vi "Filter Wheel GUI.vi"(9 "Standalone":bool=TRUE, 10 "Init Data":variant, 11 "Filter Wheel name":string="Default") -> ()   [LabVIEW 2024]
uses:
  Filter Wheel Arduino Control/Filter Wheel Arduino Command cluster.ctl
  typedefs/CC enum Operation Mode.ctl
  Filter Wheel Arduino Control/Filter Wheel Arduino Homing cluster.ctl
  Filter Wheel Object/Filter Wheel.lvclass
  Filter Wheel configuration.ctl
  Filter Wheel Object/Filter Wheel Details.ctl
  Subsystems/SS typedef cluster Instrument Command Queue Data.ctl
  Subsystems/SS cluster Data Queue type.ctl
  FW cmd Q Move Parameters.ctl
  <vilib>/Utility/miscctls.llb/LVRowAndColumnTypeDef.ctl
  FW cluster Status.ctl
  FW enum status.ctl
  Filter Wheel Object/Filter Wheel.lvclass/Filter Wheel.ctl
  hk-channel-class/hk-channel-class/HK Item/HK Channel Units and Setup.ctl
  hk-channel-class/hk-channel-class/HK Item/HK Channel enum Data Type.ctl
  hk-channel-class/hk-channel-class/HK Item/HK Item.lvclass
  hk-channel-class/hk-channel-class/HK Item/HK Channel cluster Telemetry Data.ctl
  FW cmd Q Move Position Parameters.ctl
  typedefs/CC cluster Alarm Data.ctl
  Filter Wheel Simulator/Filter Wheel Simulator.lvclass
  C:/Development/Prime-RIMAS/Filter Wheel/Filter Wheel Object/Filter Wheel.lvclass
  Filter Wheel Simulator/Filter Wheel Simulator.lvclass/Filter Wheel Simulator.ctl
  Filter Wheel Arduino Control/FW Arduino Control.lvclass
panel:
  out "Messages":string
  in  "Mode":T1
  in  "Tab Control":T2(tab)
  out "Wheel Name":string
  out "Moving Message":string="Filter Wheel Moving...."
  in  "Error":bool
  out "Homed":bool[](array[boolean])
  in  "Wheel To Home":u16(ring)
  in  "STOP":bool
  out "Connected":bool
  in  "Filter Wheel Displays":T3 {"Gauge 0" scale=0.0..3.0; "Gauge 4" scale=0.0..7.0; "Gauge 3" scale=0.0..5.0; "Gauge 2" scale=0.0..3.0; "Gauge 5" scale=0.0..32768.0; "Gauge 8" scale=0.0..32768.0; "Gauge 6" scale=0.0..32768.0; "Gauge 7" scale=0.0..32768.0}
  in  "Home":bool
  in  "Alarms?":bool=TRUE
  in  "Default Speed":u16=200 min=20 max=4000 step=10
  in  "Movement Parameters":T4
  in  "Sim Velocity (steps/sec)":i32
  in  "Connect":bool
  in  "Serial Port":refnum<visa-resource-name>="COM11"
  in  "Simulate":bool
  in  "Close":bool
  in  "Filter Wheel Table":cluster{i32[], "Dir":bool}[][](array[cluster])=[[{[], "Dir"=TRUE}, {[2800], "Dir"=TRUE}, {[2800, 2800], "Dir"=TRUE}, {[950, 1850], "Dir"=FALSE}], [{[2800], "Dir"=FALSE}, {[], "Dir"=TRUE}, {[2800], "Dir"=TRUE}, {[2800, 2800], "Dir"=TRUE}], [{[2800, 2800], "Dir"=FALSE}, {[2800], "Dir"=FALSE}, {[], "Dir"=TRUE}, {[2800], "Dir"=TRUE}], [{[2800, 2800], "Dir"=TRUE}, {[2800, 2800], "Dir"=FALSE}, {[2800], "Dir"=FALSE}, {[], "Dir"=TRUE}]]
  in  "Open Arduino Log":bool
  out "Moving":bool[](array[boolean])
  out "Last Move Positions":u32[](array[numeric])
  out "On the notch":bool[](array[boolean])
  in  "Filter Wheel Settings":T5={"Direction"=TRUE, "NUMBER OF  STEPS"=2900, "SPEED STEPS/SEC"=200, "ACC/DECEL STEPS/SEC^2"=4000, "Move mode"=0, "EN/DIS?"=TRUE, "delay before \nread (ms)"=750, "Timeout before \nstop (ms)"=13000} {"Move mode" items=["Relative steps ##", "Search switch"]; "ACC/DECEL STEPS/SEC^2" max=4000; "SPEED STEPS/SEC" min=20 max=4000 step=10}
  in  "MOTOR NUMBER":u8 max=3 step=1
  in  "Command Preview":string
  out "Response":string
  in  "Send Command":bool
  in  "Read":bool
  in  "Focus Offsets":string[][](table)
  in  "Restore Defaults":bool
  in  "Remove Pos":bool
  in  "Add Pos":bool
  in  "Save Button":bool
  in  "Remove Fw":bool
  in  "Add Fw":bool
  in  "Wheels":i32(listbox)
  in  "Positions":i32(listbox)
  # "Click for info"
  # "Enter the combined offset of each combination of filters."
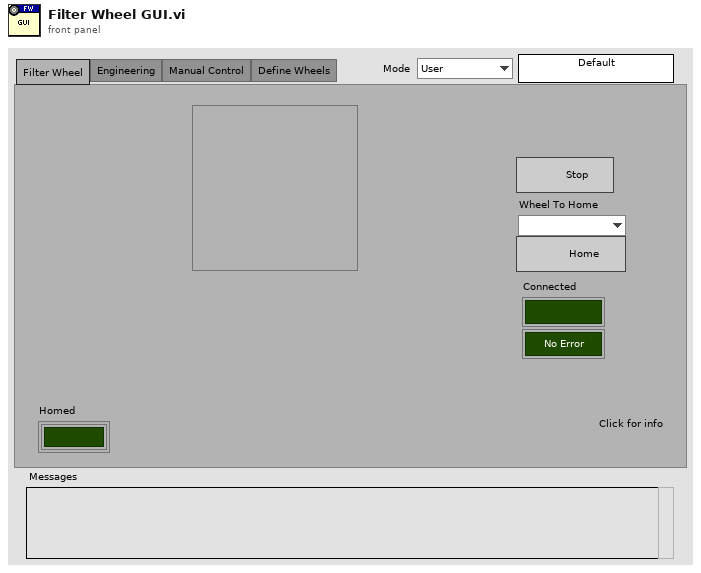
[diagram p1: front panel]
types:
  T1 = typedef "CC enum Operation Mode.ctl" = enum16{"User", "Engineering"}
  T2 = enum32{"Filter Wheel", "Engineering", "Manual Control", "Define Wheels"}
  T3 = cluster{"Gauge 0":i32, "Gauge 2":i32, "Gauge 3":i32, "Gauge 4":i32, "Gauge 5":i32, "Gauge 6":i32, "Gauge 7":i32, "Gauge 8":i32, "Position 0":i32, "Position 1":i32, "Position 2":i32, "Position 3":i32}
  T4 = typedef "Filter Wheel Arduino Homing cluster.ctl" = cluster{"Direction (F: CW)":bool, "Speed":i32, "Accel":i32, "Min Distance":i32, "Short Leg":i32, "Error Cnts":i32}
  T5 = typedef "Filter Wheel Arduino Command cluster.ctl" = cluster{"Direction":bool, "NUMBER OF  STEPS":u32, "SPEED STEPS/SEC":u16, "ACC/DECEL STEPS/SEC^2":u16, "Move mode":u16, "EN/DIS?":bool, "delay before \nread (ms)":u32, "Timeout before \nstop (ms)":u32}
  T6 = typedef "SS typedef cluster Instrument Command Queue Data.ctl" = cluster{"Cmd":string, "Parameters":variant}
  T7 = typedef "Filter Wheel.lvclass/Filter Wheel configuration.ctl" = cluster{"Num Wheels":i32, "Filters":T8[], "Invalid Combinations":i32[][], "Addr":refnum<visa-resource-name>, "Name":string, "Simulate":bool, "Homing Parameters":T4, "Default Speed":u16}
  T8 = typedef "Filter Wheel.lvclass/Filter Wheel Details.ctl" = cluster{"Names":string[], "Relative Position":i32[], "Wheel Name":string}
  T9 = typedef "FW cmd Q Move Parameters.ctl" = cluster{"Wheel ID":i32, "Position":i32}
  T10 = typedef "LVRowAndColumnTypeDef.ctl" = cluster{"Row":i32, "Column":i32}
  T11 = typedef "FW cluster Status.ctl" = cluster{"State":T12, "Positions":i32[], "Names":string[], "Notch":bool[], "Moving":bool[]}
  T12 = typedef "FW enum status.ctl" = enum16{"Initializing", "Moving", "Move Complete", "Error"}
  T13 = cluster{"state":refnum<user-event>, "Filter Wheel ref":refnum<class "Filter Wheel.lvclass">, "Filter Wheel Info":T7, "FW names":string[], "Pos Names":cluster{"Table":string[][]}[], "cmd q":refnum<queue>, "Cmd":T6, "Data Q":refnum<queue>, "Move":T9, "error":errorcluster, "next poll":timestamp, "FW refs":refnum<vi>[], "Wheel":i32, "Coords":T10, "Motor #":u8, "fw name":string, "Simulate":bool, "ch names":string[][], "FW Status":T11, "Error State":string, "Name":string, "Period":dbl}
  T14 = typedef "HK Item.lvclass/HK Channel Units and Setup.ctl" = cluster{"Unit Type":string, "Units":string, "Configuration":string, "Digits":i32, "Data Type":T15, "Exponential?":bool, "Source":string}
  T15 = typedef "HK Item.lvclass/HK Channel enum Data Type.ctl" = enum16{"Floating Point", "Integer", "Enum", "String", "Waveform", "File"}
  T16 = typedef "SS cluster Data Queue type.ctl" = cluster{"Source":string, "Type":string, "Data":variant}
  T17 = typedef "FW cmd Q Move Position Parameters.ctl" = cluster{"Position Names":string[]}
  T18 = enum32{"Page Enabled", "Page Disabled", "Page Disabled & Grayed"}
  T19 = typedef "CC cluster Alarm Data.ctl" = cluster{"Measured Value":dbl, "Alarm Low":dbl, "Alarm High":dbl, "Message":string, "Source":string}
  T20 = typedef "HK Item.lvclass/HK Channel cluster Telemetry Data.ctl" = cluster{"Ch Names":string[], "Ch Values":dbl[], "Timestamp":timestamp, "Data Type":T15}
  T21 = cluster{"Gauge 0":bool, "Gauge 2":bool, "Gauge 3":bool, "Gauge 4":bool, "Gauge 5":bool, "Gauge 6":bool, "Gauge 7":bool, "Gauge 8":bool, "Position 0":bool, "Position 1":bool, "Position 2":bool, "Position 3":bool}
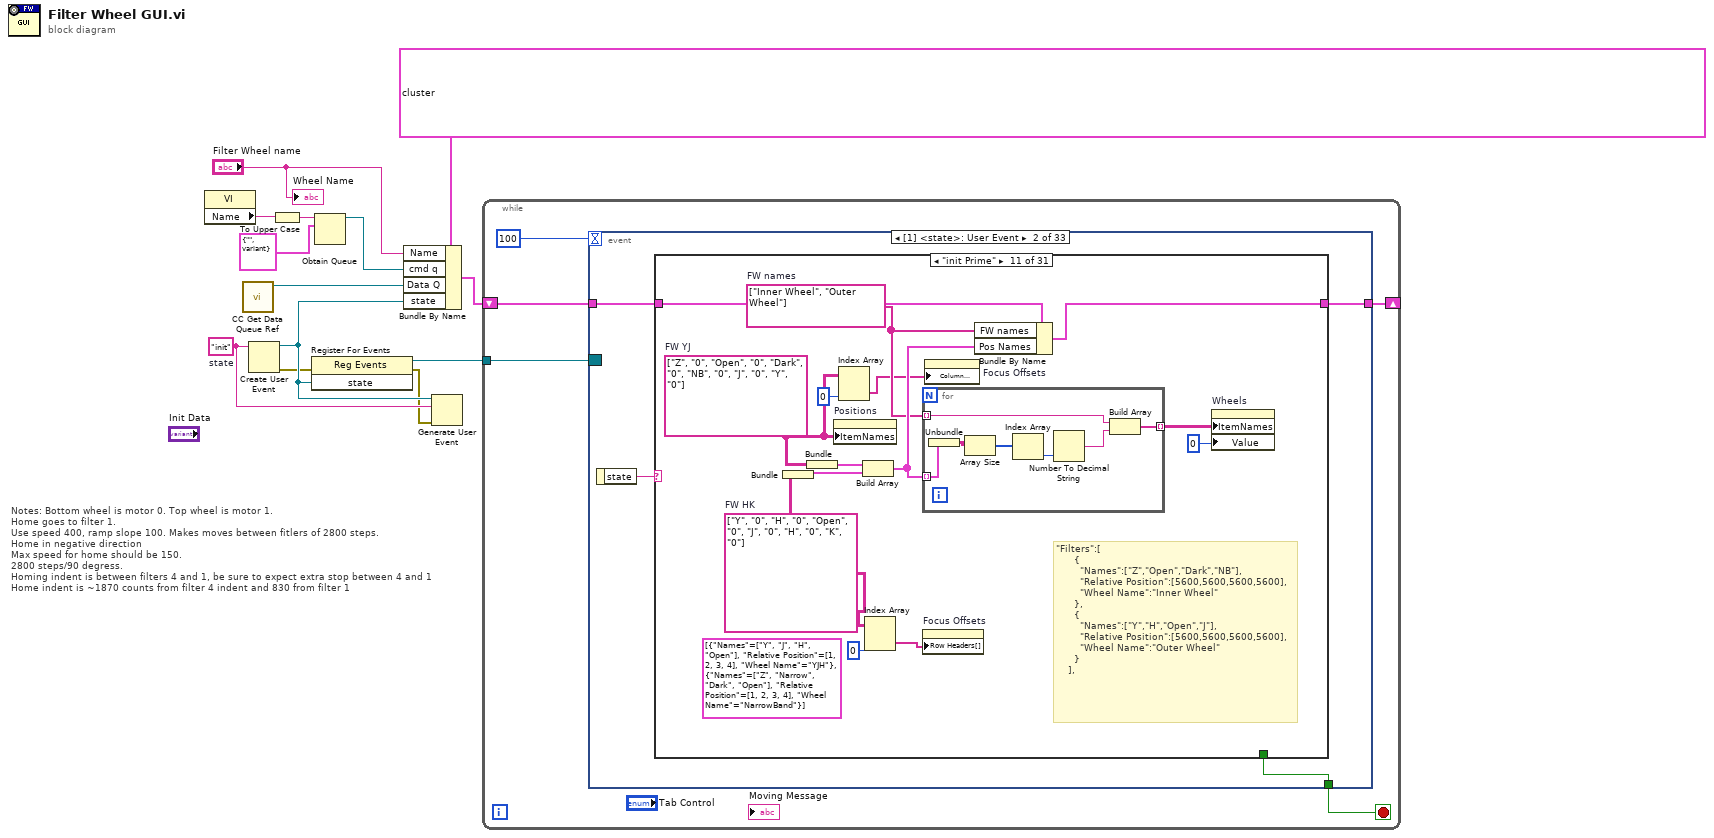
[diagram p0: block diagram]
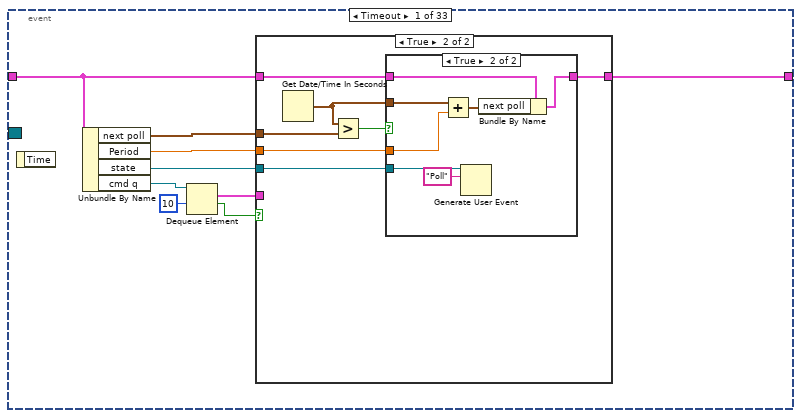
[diagram p2: hidden frame]
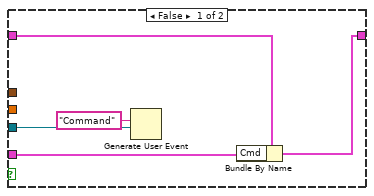
[diagram p3: hidden frame]
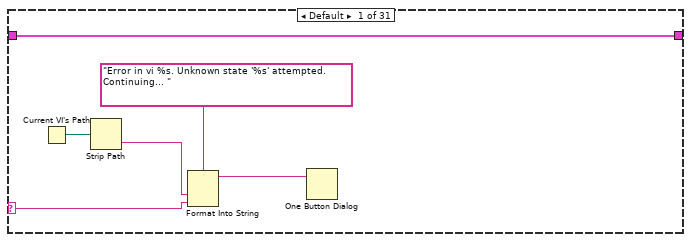
[diagram p5: hidden frame]
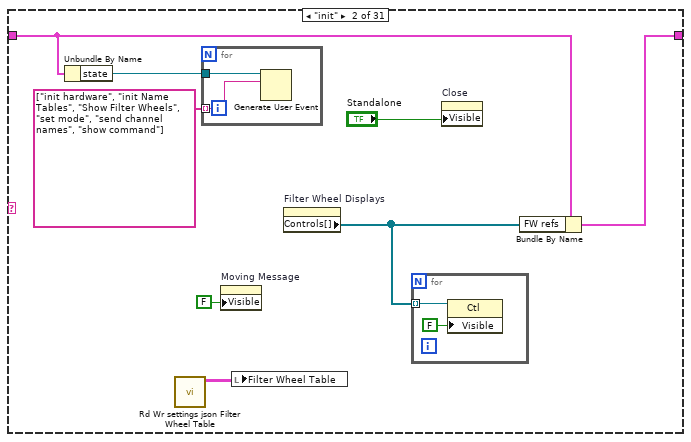
[diagram p6: hidden frame]
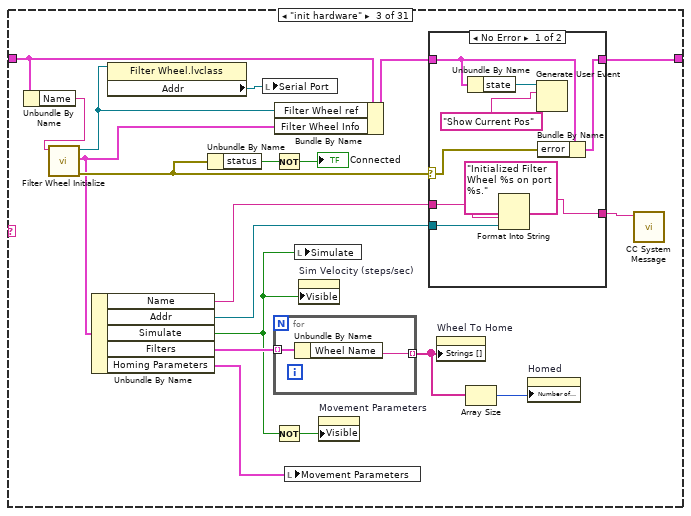
[diagram p7: hidden frame]
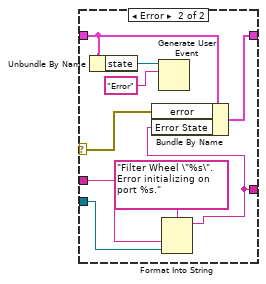
[diagram p8: hidden frame]
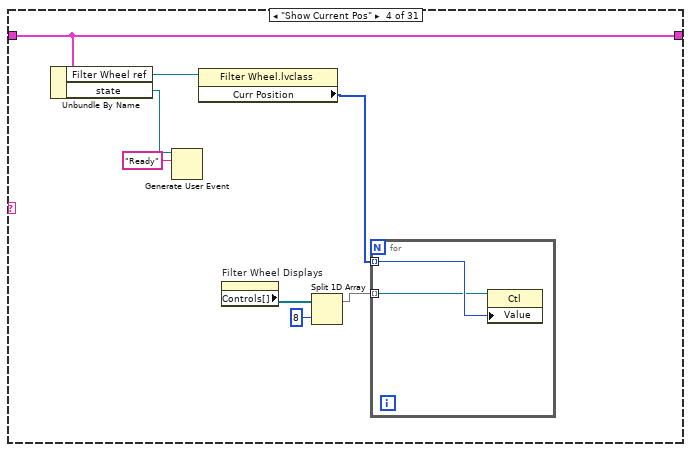
[diagram p9: hidden frame]
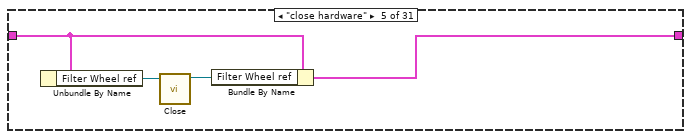
[diagram p10: hidden frame]
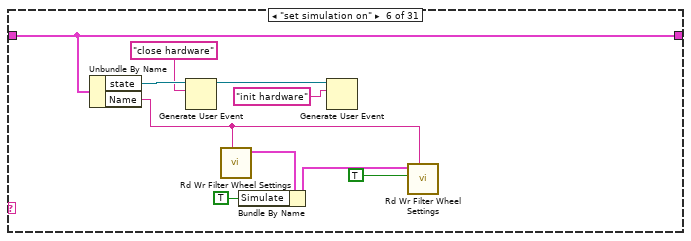
[diagram p11: hidden frame]
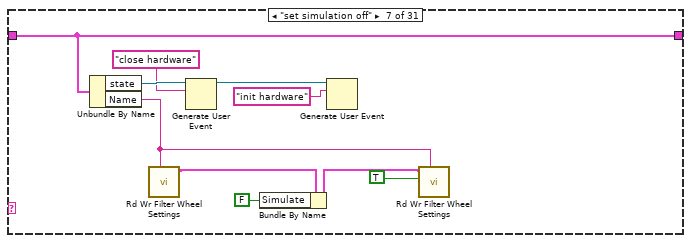
[diagram p12: hidden frame]
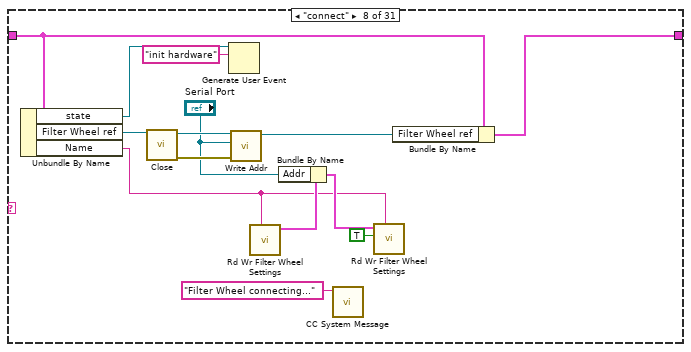
[diagram p13: hidden frame]
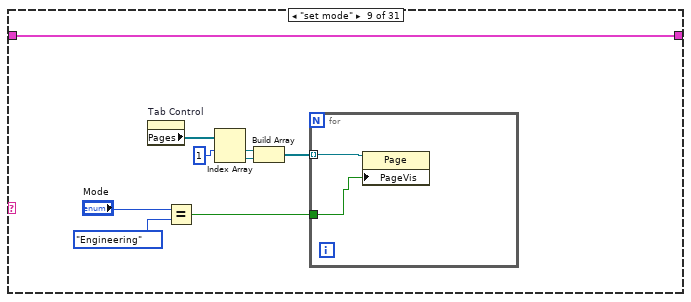
[diagram p14: hidden frame]
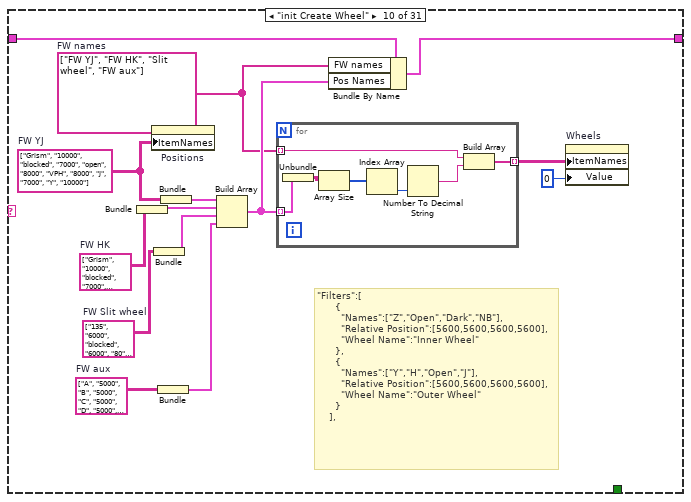
[diagram p15: hidden frame]
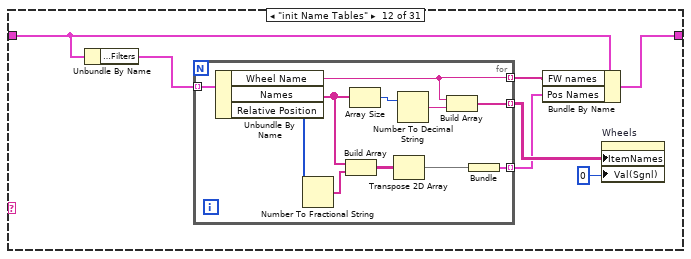
[diagram p16: hidden frame]
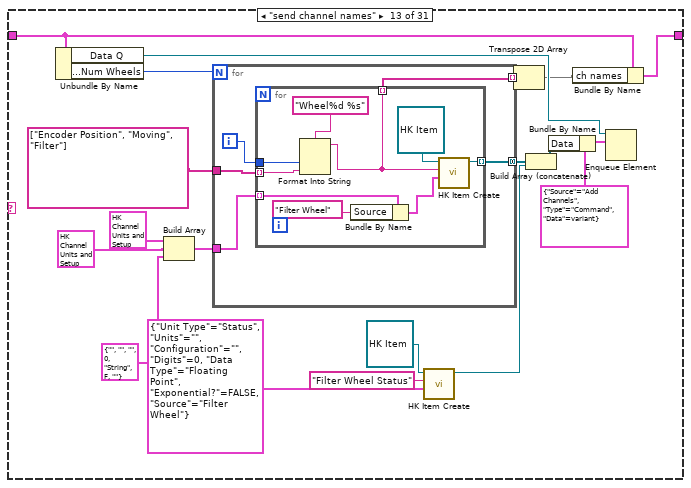
[diagram p17: hidden frame]
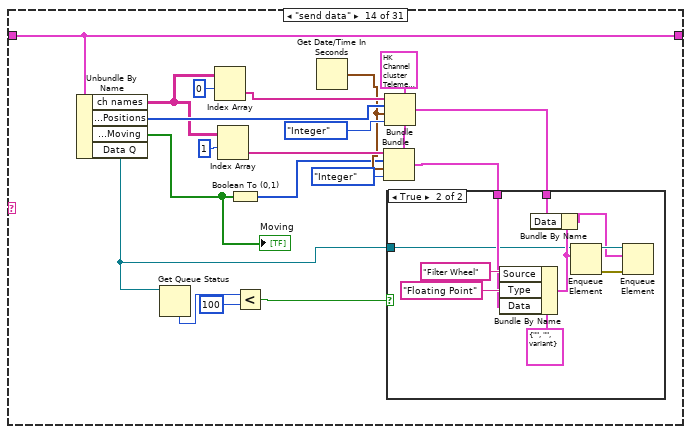
[diagram p18: hidden frame]
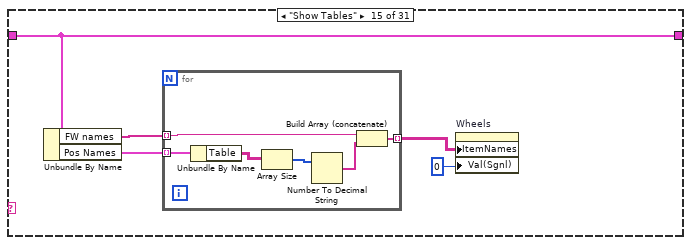
[diagram p20: hidden frame]
diagram:
  w9 = "init"  # state
  # "Notes: Bottom wheel is motor 0. Top wheel is motor 1.\nHome goes to filter 1. \nUse speed 400, ramp slope 100. Makes moves between fitlers of 2800 steps.\nHome in negative direction\nMax speed for home should be 150.\n2800 steps/90 degress.\nHoming indent is between filters 4 and 1, be sure to expect extra stop between 4 and 1\nHome indent is ~1870 counts from filter 4 indent and 830 from filter 1"
  n1 = property class="VI"() -> ("Name"=w5:string)  [unwired: 2 in, 2 out]
  n2 = call "CC Get Data Queue Ref.vi"() -> ("Data Q"=w6:refnum<queue>)  [unwired: 10 in, 1 out]
  n3 = Create User Event(user event datatype=w9) -> (user event=w11:refnum<user-event>, error out=w7:errorcluster)  [unwired: 1 in]
  n4 = To Upper Case(1:w5) -> (0:w4:string)
  n5 = register-events(error in=w7, w11) -> (reference out=w10:refnum<event-registration>, error out=w8:errorcluster)  [unwired: 1 in]
  n6 = Obtain Queue(name (unnamed)=w4, element data type=T6 {"Cmd"="", "Parameters"=variant}) -> (queue out=w2:refnum<queue>)  [unwired: 3 in, 2 out]
  n7 = Bundle By Name(cluster=T13 {"state"=refnum, "Filter Wheel ref"=refnum, "Filter Wheel Info"={"Num Wheels"=0, "Filters"=[], "Invalid Combinations"=[], "Addr"="", "Name"="", "Simulate"=FALSE, "Homing Parameters"={"Direction (F: CW)"=TRUE, "Speed"=150, "Accel"=400, "Min Distance"=2700, "Short Leg"=0, "Error Cnts"=0}, "Default Speed"=1000}, "FW names"=["FW YJ", "FW HK", "Slit wheel", "FW aux"], "Pos Names"=[], "cmd q"=refnum, "Cmd"={"Cmd"="", "Parameters"=variant}, "Data Q"=refnum, "Move"={"Wheel ID"=0, "Position"=0}, "error"={"status"=FALSE, "code"=0, "source"=""}, "next poll"=timestamp(0 s since 1904-01-01), "FW refs"=[], "Wheel"=0, "Coords"={"Row"=0, "Column"=0}, "Motor #"=0, "fw name"="", "Simulate"=TRUE, "ch names"=[], "FW Status"={"State"=enum."Move Complete", "Positions"=[], "Names"=[], "Notch"=[], "Moving"=[FALSE, FALSE]}, "Error State"="", "Name"="PRIME", "Period"=1.0}, "Name"="Filter Wheel name", "cmd q"=w2, "Data Q"=w6, "state"=w11) -> (w12:T13)
  n8 = Generate User Event(user event=w11, event data cluster=w9, error in=w8) -> ()  [unwired: 1 in, 2 out]
  n9 = while {
    tunnel: w10 -> [w18]
    shift-right: [w17] -> _
    shift-left: w12 -> [w14]
    stop <- w16 stop-if-true
    n10 = event shown="[1] <state>: User Event" {
      selector: w18 -> [_ _ _ _ _ _ _ _ _ _ _ _ _ _ _ _ _ _ _ _ _ _ _ _ _ _ _ _ _ _ _ _ _]
      dyn-events: _ -> [_ _ _ _ _ _ _ _ _ _ _ _ _ _ _ _ _ _ _ _ _ _ _ _ _ _ _ _ _ _ _ _ _]
      timeout: 100 -> [_ _ _ _ _ _ _ _ _ _ _ _ _ _ _ _ _ _ _ _ _ _ _ _ _ _ _ _ _ _ _ _ _]
      tunnel: w14 -> [w22 w50 w587 w589 w598 w604 w607 w610 w612 w634 w641 w650 w656 w657 w672 w675 w678 w679 w684 w687 w696 w700 w706 w713 w718 w734 w756 w765 w771 w794 w805 w825 w829]
      tunnel: [w21 w49 w587 w588 w598 w604 w607 w610 w615 w635 w642 w650 w656 w658 w672 w675 w678 w680 w684 w687 w697 w701 w707 w714 w719 w735 w757 w766 w772 w795 w806 w825 w829] -> w17
      tunnel: [_ w48 _ _ _ _ _ _ _ _ _ _ _ _ _ _ _ _ _ _ _ _ _ _ _ _ _ _ _ _ _ _ _] -> w16
      event Timeout {
        n11 = event-data() -> ()  [unwired: 1 in, 1 out]
        n12 = Unbundle By Name(w22) -> ("next poll"=w20:timestamp, "Period"=w19:dbl, "state"=w23:refnum<user-event>, "cmd q"=w27:refnum<queue>)
        n13 = Dequeue Element(queue=w27, timeout in ms (-1)=10) -> (element=w24:T6, timed out?=w25:bool)  [unwired: 1 in, 2 out]
        n14 = case shown="True" w25 {
          tunnel: w24 -> [w29 _]
          tunnel: w23 -> [w32 w36]
          tunnel: w22 -> [w30 w37]
          tunnel: [w28 w34] -> w21
          tunnel: w20 -> [_ w39]
          tunnel: w19 -> [_ w33]
          frame False {
            n15 = Generate User Event(user event=w32, event data cluster="Command" ("event data")) -> ()  [unwired: 2 in, 2 out]
            n16 = Bundle By Name(cluster=w30, "Cmd"=w29) -> (w28:T13)
          }
          frame True {
            n17 = Get Date/Time In Seconds() -> (seconds since 1Jan1904=w35:timestamp)
            n18 = Greater?(x=w35, y=w39) -> (0:w38:bool)
            n19 = case shown="True" w38 {
              tunnel: w37 -> [w40 w47]
              tunnel: w36 -> [_ w46]
              tunnel: w35 -> [_ w45]
              tunnel: [w40 w43] -> w34
              tunnel: w33 -> [_ w41]
              frame False {
              }
              frame True {
                n20 = Add(x=w45, y=w41) -> (x+y=w44:timestamp)
                n21 = Generate User Event(user event=w46, event data cluster="Poll" ("event data")) -> ()  [unwired: 2 in, 2 out]
                n22 = Bundle By Name(cluster=w47, "next poll"=w44) -> (w43:T13)
              }
            }
          }
        }
      }
      event User Event {
        n23 = event-data() -> ("state"=w51:string)  [unwired: 1 in]
        n24 = case shown="\"init Prime\"" w51 {
          selector: w51 -> [w56 _ _ _ _ _ _ _ _ _ _ _ _ _ _ _ _ _ _ _ _ _ _ _ _ _ _ _ _ _ _]
          tunnel: w50 -> [w52 w64 w75 w116 w119 w131 w141 w152 w165 w168 w195 w214 w235 w279 w294 w312 w328 w337 w379 w437 w460 w488 w504 w517 w533 w541 w548 w555 w560 w581 w584]
          tunnel: [w52 w65 w87 w116 w120 w131 w141 w153 w165 w169 w196 w215 w236 w279 w294 w312 w328 w338 w388 w438 w478 w487 w505 w518 w534 w542 w548 w555 w561 w581 w584] -> w49
          tunnel: [_ _ _ _ _ _ _ _ _ _ _ _ _ _ _ _ _ _ _ _ _ _ _ _ _ _ _ _ _ _ TRUE] -> w48
          frame Default {
            n25 = Current VI's Path() -> (path=w55:path)
            n26 = Strip Path(path=w55) -> (name=w54:string)  [unwired: 1 out]
            n27 = Format Into String(format string="Error in vi %s. Unknown state '%s' attempted. Continuing... ", w54, w56) -> (resulting string=w53:string)  [unwired: 2 in, 1 out]
            n28 = One Button Dialog(message=w53) -> ()  [unwired: 1 in, 1 out]
          }
          frame "init" {
            n29 = Unbundle By Name(w64) -> ("state"=w63:refnum<user-event>)
            n30 = call "Rd Wr settings json Filter Wheel Table.vi"() -> ("Filter Wheel Table"=w58:cluster{i32[], bool}[][])  [unwired: 10 in, 1 out]
            n31 = for {
              tunnel: w63 -> [w69]
              tunnel: string[] ["init hardware", "init Name Tables", "Show Filter Wheels", "set mode", "send channel names", "show command"] -> [w68] mode=indexing
              n32 = Generate User Event(user event=w69, event data cluster=w68) -> ()  [unwired: 2 in, 2 out]
            }
            n33 = property on="Moving Message" class="Str"("Visible"=FALSE) -> ()  [unwired: 2 in, 2 out]
            n34 = local write "Filter Wheel Table"(w58) -> ()
            n35 = property on="Filter Wheel Displays" class="Clust (strict)"() -> ("Controls[]"=w60:refnum<vi>[])  [unwired: 2 in, 2 out]
            n36 = for {
              tunnel: w60 -> [w67] mode=indexing
              n37 = property class="Ctl"(reference=w67, "Visible"=FALSE) -> ()  [unwired: 1 in, 2 out]
            }
            n38 = property on="Close" class="Bool"("Visible"="Standalone") -> ()  [unwired: 2 in, 2 out]
            n39 = Bundle By Name(cluster=w64, "FW refs"=w60) -> (w65:T13)
          }
          frame "init hardware" {
            n40 = Unbundle By Name(w75) -> ("Name"=w74:string)
            n41 = call "Filter Wheel Initialize.vi"("Wheel Name"=w74) -> ("error out"=w86:errorcluster, "Filter Wheel Info"=w83:T7, "Filter Wheel.lvclass"=w71:refnum<class "Filter Wheel.lvclass">)  [unwired: 8 in]
            n42 = Unbundle By Name(w83) -> ("Name"=w82:string, "Addr"=w81:refnum<visa-resource-name>, "Simulate"=w72:bool, "Filters"=w79:T8[], "Homing Parameters"=w78:T4)
            n43 = property class="Filter Wheel.lvclass"(reference=w71) -> ("Addr"=w70:refnum<visa-resource-name>)  [unwired: 1 in, 2 out]
            n44 = Unbundle By Name(w86) -> ("status"=w85:bool)
            n45 = local write "Serial Port"(w70) -> ()
            n46 = Not(x=w85) -> (.not. x?=→"Connected":bool)
            n47 = for {
              tunnel: [w89] -> w77 mode=indexing
              tunnel: w79 -> [w90] mode=indexing
              n48 = Unbundle By Name(w90) -> ("Wheel Name"=w89:string)
            }
            n49 = Not(x=w72) -> (.not. x?=w73:bool)
            n50 = Bundle By Name(cluster=w75, "Filter Wheel ref"=w71, "Filter Wheel Info"=w83) -> (w88:T13)
            n51 = local write "Movement Parameters"(w78) -> ()
            n52 = local write "Simulate"(w72) -> ()
            n53 = property on="Sim Velocity (steps/sec)" class="DigNum (strict)"("Visible"=w72) -> ()  [unwired: 2 in, 2 out]
            n54 = property on="Movement Parameters" class="Clust (strict)"("Visible"=w73) -> ()  [unwired: 2 in, 2 out]
            n55 = case shown="No Error" w86 {
              selector: w86 -> [w93 w107]
              tunnel: [w92 w106] -> w87
              tunnel: w88 -> [w91 w105]
              tunnel: w82 -> [w98 w102]
              tunnel: w81 -> [w97 w101]
              tunnel: [w96 w100] -> w80
              frame No Error {
                n56 = Unbundle By Name(w91) -> ("state"=w94:refnum<user-event>)
                n57 = Format Into String(format string="Initialized Filter Wheel %s on port %s.", w98, w97) -> (resulting string=w96:string)  [unwired: 2 in, 1 out]
                n58 = Generate User Event(user event=w94, event data cluster="Show Current Pos" ("event data")) -> ()  [unwired: 2 in, 2 out]
                n59 = Bundle By Name(cluster=w91, "error"=w93) -> (w92:T13)
              }
              frame Error {
                n60 = Unbundle By Name(w105) -> ("state"=w104:refnum<user-event>)
                n61 = Generate User Event(user event=w104, event data cluster="Error" ("event data")) -> ()  [unwired: 2 in, 2 out]
                n62 = Format Into String(format string="Filter Wheel \"%s\". Error initializing on port %s.", w102, w101) -> (resulting string=w100:string)  [unwired: 2 in, 1 out]
                n63 = Bundle By Name(cluster=w105, "error"=w107, "Error State"=w100) -> (w106:T13)
              }
            }
            n64 = property on="Wheel To Home" class="Ring (strict)"("Strings []"=w77) -> ()  [unwired: 2 in, 2 out]
            n65 = Array Size(array=w77) -> (size(s)=w76:i32)
            n66 = property on="Homed" class="Arr (strict)"("Number of Columns"=w76) -> ()  [unwired: 2 in, 2 out]
            n67 = call "CC System Message.vi"("Message"=w80) -> ()  [unwired: 10 in, 1 out]
          }
          frame "Show Current Pos" {
            n68 = Unbundle By Name(w116) -> ("Filter Wheel ref"=w115:refnum<class "Filter Wheel.lvclass">, "state"=w114:refnum<user-event>)
            n69 = Generate User Event(user event=w114, event data cluster="Ready" ("event data")) -> ()  [unwired: 2 in, 2 out]
            n70 = property class="Filter Wheel.lvclass"(reference=w115) -> ("Curr Position"=w110:i32[])  [unwired: 1 in, 2 out]
            n71 = property on="Filter Wheel Displays" class="Clust (strict)"() -> ("Controls[]"=w112:refnum<vi>[])  [unwired: 2 in, 2 out]
            n72 = Split 1D Array(array=w112, index=8) -> (first subarray=w109:refnum<vi>[])  [unwired: 1 out]
            n73 = for {
              tunnel: w110 -> [w118] mode=indexing
              tunnel: w109 -> [w117] mode=indexing
              n74 = property class="Ctl"(reference=w117, "Value"=w118) -> ()  [unwired: 1 in, 2 out]
            }
          }
          frame "close hardware" {
            n75 = Unbundle By Name(w119) -> ("Filter Wheel ref"=w122:refnum<class "Filter Wheel.lvclass">)
            n76 = call-dynamic "Close.vi"("Filter Wheel in"=w122) -> ("Filter Wheel out"=w121:refnum<class "Filter Wheel.lvclass">)  [unwired: 9 in, 1 out]
            n77 = Bundle By Name(cluster=w119, "Filter Wheel ref"=w121) -> (w120:T13)
          }
          frame "set simulation on" {
            n78 = Unbundle By Name(w131) -> ("state"=w130:refnum<user-event>, "Name"=w123:string)
            n79 = Generate User Event(user event=w130, event data cluster="close hardware" ("event data")) -> (user event out=w129:refnum<user-event>)  [unwired: 2 in, 1 out]
            n80 = call "Rd Wr Filter Wheel Settings.vi"("Wheel Name"=w123) -> ("Filter Wheel Settings"=w126:T7)  [unwired: 9 in, 1 out]
            n81 = Bundle By Name(cluster=w126, "Simulate"=TRUE) -> (w125:T7)
            n82 = Generate User Event(user event=w129, event data cluster="init hardware" ("event data")) -> ()  [unwired: 2 in, 2 out]
            n83 = call "Rd Wr Filter Wheel Settings.vi"("Wheel Name"=w123, "Write? (F:Read)"=TRUE, "Filter Wheel Settings"=w125) -> ()  [unwired: 7 in, 2 out]
          }
          frame "set simulation off" {
            n84 = Unbundle By Name(w141) -> ("state"=w140:refnum<user-event>, "Name"=w133:string)
            n85 = call "Rd Wr Filter Wheel Settings.vi"("Wheel Name"=w133) -> ("Filter Wheel Settings"=w136:T7)  [unwired: 9 in, 1 out]
            n86 = Generate User Event(user event=w140, event data cluster="close hardware" ("event data")) -> (user event out=w139:refnum<user-event>)  [unwired: 2 in, 1 out]
            n87 = Bundle By Name(cluster=w136, "Simulate"=FALSE) -> (w135:T7)
            n88 = Generate User Event(user event=w139, event data cluster="init hardware" ("event data")) -> ()  [unwired: 2 in, 2 out]
            n89 = call "Rd Wr Filter Wheel Settings.vi"("Wheel Name"=w133, "Write? (F:Read)"=TRUE, "Filter Wheel Settings"=w135) -> ()  [unwired: 7 in, 2 out]
          }
          frame "connect" {
            n90 = Unbundle By Name(w152) -> ("state"=w150:refnum<user-event>, "Filter Wheel ref"=w156:refnum<class "Filter Wheel.lvclass">, "Name"=w143:string)
            n91 = call-dynamic "Close.vi"("Filter Wheel in"=w156) -> ("error out"=w154:errorcluster, "Filter Wheel out"=w155:refnum<class "Filter Wheel.lvclass">)  [unwired: 9 in]
            n92 = Generate User Event(user event=w150, event data cluster="init hardware" ("event data")) -> ()  [unwired: 2 in, 2 out]
            n93 = call "Write Addr.vi"("error in (no error)"=w154, "Addr"="Serial Port", "Filter Wheel in"=w155) -> ("Filter Wheel out"=w151:refnum<class "Filter Wheel.lvclass">)  [unwired: 7 in, 1 out]
            n94 = call "Rd Wr Filter Wheel Settings.vi"("Wheel Name"=w143) -> ("Filter Wheel Settings"=w148:T7)  [unwired: 9 in, 1 out]
            n95 = Bundle By Name(cluster=w148, "Addr"="Serial Port") -> (w146:T7)
            n96 = call "CC System Message.vi"("Message"="Filter Wheel connecting...") -> ()  [unwired: 10 in, 1 out]
            n97 = call "Rd Wr Filter Wheel Settings.vi"("Wheel Name"=w143, "Write? (F:Read)"=TRUE, "Filter Wheel Settings"=w146) -> ()  [unwired: 7 in, 2 out]
            n98 = Bundle By Name(cluster=w152, "Filter Wheel ref"=w151) -> (w153:T13)
          }
          frame "set mode" {
            n99 = property on="Tab Control" class="TabCtl (strict)"() -> ("Pages"=w164:refnum<vi>[])  [unwired: 2 in, 2 out]
            n100 = Equal?(x="Mode", y=CC_enum_Operation_Mode."Engineering") -> (x = y?=w157:bool)
            n101 = Index Array(array=w164, index #1=1 ("index")) -> (element #1=w162:refnum<vi>, element #2=w161:refnum<vi>)  [unwired: 1 in]
            n102 = Build Array(w162, w161) -> (w160:refnum<vi>[])
            n103 = for {
              tunnel: w160 -> [w167] mode=indexing
              tunnel: w157 -> [w166]
              n104 = property class="Page"(reference=w167, "PageVis"=w166) -> ()  [unwired: 1 in, 2 out]
            }
          }
          frame "init Create Wheel" {
            w170 = string[] ["FW YJ", "FW HK", "Slit wheel", "FW aux"]  # FW names
            w178 = string[][] [["Grism", "10000"], ["blocked", "7000"], ["open", "8000"], ["VPH", "8000"], ["J", "7000"], ["Y", "10000"]]  # FW YJ
            w181 = string[][] [["Grism", "10000"], ["blocked", "7000"], ["open", "8000"], ["VPH", "8000"], ["H", "7000"], ["K", "10000"]]  # FW HK
            w173 = string[][] [["135", "6000"], ["blocked", "6000"], ["80", "7000"], ["open 1", "7000"], ["250", "7000"], ["open", "7000"]]  # FW Slit wheel
            w180 = string[][] [["A", "5000"], ["B", "5000"], ["C", "5000"], ["D", "5000"], ["E", "5000"], ["F", "5000"], ["G", "5000"], ["H", "5000"]]  # FW aux
            # "\"Filters\":[\n      {\n        \"Names\":[\"Z\",\"Open\",\"Dark\",\"NB\"],\n        \"Relative Position\":[5600,5600,5600,5600],\n        \"Wheel Name\":\"Inner Wheel\"\n      },\n      {\n        \"Names\":[\"Y\",\"H\",\"Open\",\"J\"],\n        \"Relative Position\":[5600,5600,5600,5600],\n        \"Wheel Name\":\"Outer Wheel\"\n      }\n    ],"
            n105 = Bundle("FW HK"=w181) -> (w175:cluster{"FW HK":string[][]})  [unwired: 1 in]
            n106 = property on="Positions" class="MCListbox (strict)"("ItemNames"=w178) -> ()  [unwired: 2 in, 2 out]
            n107 = Bundle("FW Slit wheel"=w173) -> (w174:cluster{"FW Slit wheel":string[][]})  [unwired: 1 in]
            n108 = Bundle("FW aux"=w180) -> (w172:cluster{"FW aux":string[][]})  [unwired: 1 in]
            n109 = Bundle("FW YJ"=w178) -> (w176:cluster{"FW YJ":string[][]})  [unwired: 1 in]
            n110 = Build Array(w176, w175, w174, w172) -> (w171:cluster{"FW aux":string[][]}[])
            n111 = for {
              tunnel: w171 -> [w188] mode=indexing
              tunnel: w170 -> [w184] mode=indexing
              tunnel: [w183] -> w179 mode=indexing
              n112 = Unbundle(w188) -> ("FW aux"=w182:string[][])
              n113 = Array Size(array=w182) -> (size(s)=w187:i32[])
              n114 = Index Array(array=w187) -> (element=w186:i32)  [unwired: 1 in]
              n115 = Number To Decimal String(number=w186) -> (decimal integer string=w185:string)  [unwired: 1 in]
              n116 = Build Array(w184, w185) -> (w183:string[])
            }
            n117 = Bundle By Name(cluster=w168, "FW names"=w170, "Pos Names"=w171) -> (w169:T13)
            n118 = property on="Wheels" class="MCListbox (strict)"("ItemNames"=w179, "Value"=0 ("Wheels")) -> ()  [unwired: 2 in, 2 out]
          }
          frame "init Prime" {
            (unwired) T8[] [{"Names"=["Y", "J", "H", "Open"], "Relative Position"=[1, 2, 3, 4], "Wheel Name"="YJH"}, {"Names"=["Z", "Narrow", "Dark", "Open"], "Relative Position"=[1, 2, 3, 4], "Wheel Name"="NarrowBand"}] ("Filter Wheel Info.Filters")
            w197 = string[] ["Inner Wheel", "Outer Wheel"]  # FW names
            w194 = string[][] [["Z", "0"], ["Open", "0"], ["Dark", "0"], ["NB", "0"], ["J", "0"], ["Y", "0"]]  # FW YJ
            w191 = string[][] [["Y", "0"], ["H", "0"], ["Open", "0"], ["J", "0"], ["H", "0"], ["K", "0"]]  # FW HK
            # "\"Filters\":[\n      {\n        \"Names\":[\"Z\",\"Open\",\"Dark\",\"NB\"],\n        \"Relative Position\":[5600,5600,5600,5600],\n        \"Wheel Name\":\"Inner Wheel\"\n      },\n      {\n        \"Names\":[\"Y\",\"H\",\"Open\",\"J\"],\n        \"Relative Position\":[5600,5600,5600,5600],\n        \"Wheel Name\":\"Outer Wheel\"\n      }\n    ],"
            n119 = Bundle("FW HK"=w191) -> (w199:cluster{"FW HK":string[][]})  [unwired: 1 in]
            n120 = Bundle("FW YJ"=w194) -> (w200:cluster{"FW YJ":string[][]})  [unwired: 1 in]
            n121 = property on="Positions" class="MCListbox (strict)"("ItemNames"=w194) -> ()  [unwired: 2 in, 2 out]
            n122 = Index Array(array=w194, index (col)=0 ("disabled index (col)")) -> (element=w192:string[])  [unwired: 1 in]
            n123 = Build Array(w200, w199) -> (w198:cluster{"FW HK":string[][]}[])
            n124 = Index Array(array=w191, index (col)=0 ("disabled index (col)")) -> (element=w189:string[])  [unwired: 1 in]
            n125 = for {
              tunnel: w198 -> [w209] mode=indexing
              tunnel: w197 -> [w205] mode=indexing
              tunnel: [w204] -> w202 mode=indexing
              n126 = Unbundle(w209) -> ("FW HK"=w203:string[][])
              n127 = Array Size(array=w203) -> (size(s)=w208:i32[])
              n128 = Index Array(array=w208) -> (element=w207:i32)  [unwired: 1 in]
              n129 = Number To Decimal String(number=w207) -> (decimal integer string=w206:string)  [unwired: 1 in]
              n130 = Build Array(w205, w206) -> (w204:string[])
            }
            n131 = property on="Focus Offsets" class="Tbl (strict)"("Row Headers[]"=w189) -> ()  [unwired: 2 in, 2 out]
            n132 = property on="Focus Offsets" class="Tbl (strict)"("Column Headers[]"=w192) -> ()  [unwired: 2 in, 2 out]
            n133 = Bundle By Name(cluster=w195, "FW names"=w197, "Pos Names"=w198) -> (w196:T13)
            n134 = property on="Wheels" class="MCListbox (strict)"("ItemNames"=w202, "Value"=0 ("Wheels")) -> ()  [unwired: 2 in, 2 out]
          }
          frame "init Name Tables" {
            n135 = Unbundle By Name(w214) -> ("Filter Wheel Info.Filters"=w213:T8[])
            n136 = for {
              tunnel: w213 -> [w227] mode=indexing
              tunnel: [w224] -> w212 mode=indexing
              tunnel: [w223] -> w211 mode=indexing
              tunnel: [w218] -> w210 mode=indexing
              n137 = Unbundle By Name(w227) -> ("Wheel Name"=w224:string, "Names"=w220:string[], "Relative Position"=w222:i32[])
              n138 = Number To Fractional String(number=w222) -> (F-format string=w221:string[])  [unwired: 3 in]
              n139 = Build Array(w220, w221) -> (w219:string[][])
              n140 = Array Size(array=w220) -> (size(s)=w226:i32)
              n141 = Transpose 2D Array(2D array=w219) -> (transposed array=w217:string[][])
              n142 = Number To Decimal String(number=w226) -> (decimal integer string=w225:string)  [unwired: 1 in]
              n143 = Build Array(w224, w225) -> (w223:string[])
              n144 = Bundle(w217) -> (w218:cluster{string[][]})  [unwired: 1 in]
            }
            n145 = Bundle By Name(cluster=w214, "FW names"=w212, "Pos Names"=w210) -> (w215:T13)
            n146 = property on="Wheels" class="MCListbox (strict)"("ItemNames"=w211, "Val(Sgnl)"=0 ("Wheels")) -> ()  [unwired: 2 in, 2 out]
          }
          frame "send channel names" {
            n147 = Unbundle By Name(w235) -> ("Data Q"=w239:refnum<queue>, "Filter Wheel Info.Num Wheels"=w238:i32)
            n148 = Build Array(T14 {"Unit Type"="", "Units"="Counts", "Configuration"="", "Digits"=0, "Data Type"=enum."Integer", "Exponential?"=FALSE, "Source"=""} ("Channel Setup"), T14 {"Unit Type"="", "Units"="OnOff", "Configuration"="", "Digits"=0, "Data Type"=enum."Integer", "Exponential?"=FALSE, "Source"=""} ("Channel Setup"), T14 {"Unit Type"="", "Units"="", "Configuration"="", "Digits"=0, "Data Type"=enum."String", "Exponential?"=FALSE, "Source"=""} ("Channel Setup")) -> (w242:T14[])
            n149 = for {
              N: w238 -> [_]
              tunnel: string[] ["Encoder Position", "Moving", "Filter"] -> [w251]
              tunnel: w242 -> [w250]
              tunnel: [w249] -> w237 mode=concatenating
              tunnel: [w247] -> w234 mode=indexing
              i -> [w248]
              n150 = for {
                tunnel: w251 -> [w258] mode=indexing
                tunnel: w250 -> [w253] mode=indexing
                tunnel: [w257] -> w249 mode=indexing
                tunnel: w248 -> [w256]
                tunnel: [w255] -> w247 mode=indexing
                n151 = Format Into String(format string="Wheel%d %s", w256, w258) -> (resulting string=w255:string)  [unwired: 2 in, 1 out]
                n152 = Bundle By Name(cluster=w253, "Source"="Filter Wheel") -> (w254:T14)
                n153 = call-dynamic "HK Item Create.vi"("Channel Setup"=w254, "Name"=w255, "HK Item in"=refnum<class "HK Item.lvclass"> refnum) -> ("HK Item out"=w257:refnum<class "HK Item.lvclass">)  [unwired: 7 in, 1 out]
              }
            }
            n154 = call-dynamic "HK Item Create.vi"("Channel Setup"=T14 {"Unit Type"="Status", "Units"="", "Configuration"="", "Digits"=0, "Data Type"=enum."Floating Point", "Exponential?"=FALSE, "Source"="Filter Wheel"}, "Name"="Filter Wheel Status", "HK Item in"=refnum<class "HK Item.lvclass"> refnum) -> ("HK Item out"=w228:refnum<class "HK Item.lvclass">)  [unwired: 7 in, 1 out]
            n155 = Transpose 2D Array(2D array=w234) -> (transposed array=w233:string[][])
            n156 = Build Array (concatenate)(w237, w228) -> (w229:refnum<class "HK Item.lvclass">[])
            n157 = Bundle By Name(cluster=T16 {"Source"="Add Channels", "Type"="Command", "Data"=variant} ("element"), "Data"=w229) -> (w241:T16)
            n158 = Bundle By Name(cluster=w235, "ch names"=w233) -> (w236:T13)
            n159 = Enqueue Element(queue=w239, element=w241) -> ()  [unwired: 2 in, 3 out]
          }
          frame "send data" {
            w272 = T20 {"Ch Names"=[], "Ch Values"=[], "Timestamp"=timestamp(0 s since 1904-01-01), "Data Type"=enum."Floating Point"} ("cluster")
            n160 = Unbundle By Name(w279) -> ("ch names"=w273:string[][], "FW Status.Positions"=w275:i32[], "FW Status.Moving"=w261:bool[], "Data Q"=w266:refnum<queue>)
            "Moving" <- w261
            n161 = Get Queue Status(queue=w266) -> (# elements in queue=w265:i32)  [unwired: 2 in, 7 out]
            n162 = Index Array(array=w273, index (row)=0) -> (element=w276:string[])  [unwired: 1 in]
            n163 = Index Array(array=w273, index (row)=1) -> (element=w271:string[])  [unwired: 1 in]
            n164 = Boolean To (0,1)(Boolean=w261) -> (0, 1=w262:i16[])
            n165 = Less?(x=w265, y=100) -> (x < y?=w263:bool)
            n166 = Get Date/Time In Seconds() -> (seconds since 1Jan1904=w270:timestamp)
            n167 = Bundle(cluster=w272, "Ch Names"=w271, "Ch Values"=w262, "Timestamp"=w270, "Data Type"=HK_Channel_enum_Data_Type."Integer") -> (w268:T20)
            n168 = Bundle(cluster=w272, "Ch Names"=w276, "Ch Values"=w275, "Timestamp"=w270, "Data Type"=HK_Channel_enum_Data_Type."Integer") -> (w267:T20)
            n169 = case shown="True" w263 {
              tunnel: w268 -> [_ w286]
              tunnel: w267 -> [_ w283]
              tunnel: w266 -> [_ w280]
              frame False {
              }
              frame True {
                n170 = Bundle By Name(cluster=T16 {"Source"="", "Type"="", "Data"=variant} ("element"), "Source"="Filter Wheel", "Type"="Floating Point" ("Data Type"), "Data"=w286) -> (w284:T16)
                n171 = Bundle By Name(cluster=w284, "Data"=w283) -> (w282:T16)
                n172 = Enqueue Element(queue=w280, element=w284) -> (queue out=w285:refnum<queue>, error out=w281:errorcluster)  [unwired: 2 in, 1 out]
                n173 = Enqueue Element(queue=w285, element=w282, error in (no error)=w281) -> ()  [unwired: 1 in, 3 out]
              }
            }
          }
          frame "Show Tables" {
            n174 = Unbundle By Name(w294) -> ("FW names"=w293:string[], "Pos Names"=w292:cluster{"Table":string[][]}[])
            n175 = for {
              tunnel: w293 -> [w296] mode=indexing
              tunnel: w292 -> [w300] mode=indexing
              tunnel: [w295] -> w290 mode=indexing
              n176 = Unbundle By Name(w300) -> ("Table"=w299:string[][])
              n177 = Array Size(array=w299) -> (size(s)=w298:i32[])
              n178 = Number To Decimal String(number=w298) -> (decimal integer string=w297:string[])  [unwired: 1 in]
              n179 = Build Array (concatenate)(w296, w297) -> (w295:string[])
            }
            n180 = property on="Wheels" class="MCListbox (strict)"("ItemNames"=w290, "Val(Sgnl)"=0 ("Wheels")) -> ()  [unwired: 2 in, 2 out]
          }
          frame "Show Filter Wheels" {
            w306 = 4 ("dimension size")
            (unwired) string[] ["Grism", "blocked", "VPH", "open", "J", "Y"] ("Array")
            n181 = Unbundle By Name(w312) -> ("Filter Wheel Info.Filters"=w311:T8[], "FW refs"=w310:refnum<vi>[])
            n182 = Initialize Array(0.0, w306, w306) -> (w302:dbl[][])
            n183 = call "Rd Wr settings json Filter Wheel Offsets.vi"() -> ("error out"=w305:errorcluster, "Offsets"=w303:dbl[][])  [unwired: 10 in]
            n184 = for {
              tunnel: w311 -> [w324] mode=indexing
              tunnel: w310 -> [w323] mode=indexing
              tunnel: [w318] -> w309 mode=indexing
              i -> [w314]
              w315 = TRUE ("Visible")
              n185 = Unbundle By Name(w324) -> ("Wheel Name"=w320:string, "Names"=w313:string[])
              n186 = control-ref of="Gauge 0"() -> (w321:refnum<vi>)
              n187 = To More Specific Class(target class=w321, reference=w323) -> (specific class reference=w322:refnum<vi>)  [unwired: 1 in, 1 out]
              n188 = case shown="0, Default" w314 {
                tunnel: w313 -> [w325 w326]
                frame 0, Default {
                  n189 = property on="Focus Offsets" class="Tbl (strict)"("Column Headers[]"=w325) -> ()  [unwired: 2 in, 2 out]
                }
                frame 1 {
                  n190 = property on="Focus Offsets" class="Tbl (strict)"("Row Headers[]"=w326) -> ()  [unwired: 2 in, 2 out]
                }
              }
              n191 = property class="Knob (strict)"(reference=w322, "Visible"=w315, "TextLbls[]"=w313, "Caption.Text"=w320, "Visible"=w315) -> (error out=w316:errorcluster)  [unwired: 1 in, 1 out]
              n192 = Array Size(array=w313) -> (size(s)=w319:i32)
              n193 = Number To Decimal String(number=w319) -> (decimal integer string=w317:string)  [unwired: 1 in]
              n194 = Build Array(w320, w317) -> (w318:string[])
              n195 = call <vilib>:"Clear Errors.vi"("error in (no error)"=w316) -> ()  [unwired: 5 in, 2 out]
            }
            n196 = Select(t=w302, s=w305, f=w303) -> (s? t:f=w301:dbl[][])
            n197 = Number To Fractional String(number=w301, precision (6)=i16 3) -> (F-format string=w307:string[][])  [unwired: 2 in]
            n198 = local write "Focus Offsets"(w307) -> ()
            n199 = property on="Wheels" class="MCListbox (strict)"("ItemNames"=w309) -> ()  [unwired: 2 in, 2 out]
          }
          frame "show command" {
            n200 = Unbundle By Name(w328) -> ("Motor #"=w327:u8)
            n201 = call "Arduino Generate Command String.vi"("Filter Wheel Settings"="Filter Wheel Settings", "MOTOR NUMBER"=w327) -> ("Cmd String"=w330:string)  [unwired: 9 in]
            n202 = property on="Command Preview" class="Str"("Value"=w330) -> ()  [unwired: 2 in, 2 out]
          }
          frame "Command" {
            n203 = Unbundle By Name(w337) -> ("state"=w339:refnum<user-event>, "Data Q"=w340:refnum<queue>, "Cmd.Cmd"=w335:string, "Cmd.Parameters"=w333:variant)
            n204 = Variant To Flattened String(Variant=w333) -> (data string=w334:string)  [unwired: 1 out]
            n205 = Format Into String(format string="Filter Wheel Command %s. Parameters %s" ("Message"), w335, w334) -> (resulting string=w332:string)  [unwired: 2 in, 1 out]
            n206 = call "CC System Message.vi"("Message"=w332) -> ("error out"=w331:errorcluster)  [unwired: 10 in]
            n207 = case shown="\"Move\"" w335 {
              selector: w335 -> [w350 _ _ _ _ _]
              tunnel: w340 -> [w355 _ _ _ _ _]
              tunnel: w333 -> [_ w365 w369 _ _ _]
              tunnel: w339 -> [w344 w361 _ w372 w374 w378]
              tunnel: w337 -> [w348 w356 w366 w370 w373 w376]
              tunnel: [w342 w362 w366 w370 w373 w376] -> w338
              tunnel: w331 -> [_ _ _ _ _ _]
              frame "False", Default {
                n208 = Generate User Event(user event=w344, event data cluster="Error" ("event data")) -> ()  [unwired: 2 in, 2 out]
                n209 = Format Into String(format string="Filter Wheel received invalid command. Cmd: %s", w350) -> (resulting string=w347:string)  [unwired: 2 in, 1 out]
                n210 = call "lib Quick Message Log.vi"("Message"=w350) -> ("Log"=→"Messages":string)  [unwired: 9 in, 1 out]
                n211 = Bundle By Name(cluster=T16 {"Source"="", "Type"="", "Data"=variant} ("element"), "Source"="Message" ("Data Type"), "Data"=w347) -> (w351:T16)
                n212 = Bundle By Name(cluster=w348, "Error State"="Command", "error.status"=TRUE, "error.code"=5000, "error.source"=w347) -> (w342:T13)
                n213 = Enqueue Element(queue=w355, element=w351) -> ()  [unwired: 2 in, 3 out]
              }
              frame "Move" {
                n214 = Generate User Event(user event=w361, event data cluster="Move" ("event data")) -> ()  [unwired: 2 in, 2 out]
                n215 = Get Date/Time In Seconds() -> (seconds since 1Jan1904=w358:timestamp)
                n216 = Bundle By Name(cluster=w356, "Period"=1.0, "next poll"=w358) -> (w357:T13)
                n217 = Variant To Data(type=T9 {"Wheel ID"=0, "Position"=0}, Variant=w365) -> (data=w363:T9)  [unwired: 1 in, 1 out]
                n218 = Bundle By Name(cluster=w357, "Move"=w363) -> (w362:T13)
              }
              frame "MoveFilter" {
                n219 = Variant To Data(type=T17 {"Position Names"=[]}, Variant=w369) -> (data=w367:T17)  [unwired: 1 in, 1 out]
                n220 = Unbundle By Name(w367) -> ()  [unwired: 1 out]
              }
              frame "Status" {
                n221 = Generate User Event(user event=w372, event data cluster="Send Status" ("event data")) -> ()  [unwired: 2 in, 2 out]
              }
              frame "Config" {
                n222 = Generate User Event(user event=w374, event data cluster="Send Config" ("event data")) -> ()  [unwired: 2 in, 2 out]
              }
              frame "Shutdown" {
                n223 = Generate User Event(user event=w378, event data cluster="Shutdown" ("event data")) -> ()  [unwired: 2 in, 2 out]
              }
            }
          }
          frame "Move" {
            w386 = TRUE ("Visible")
            n224 = Unbundle By Name(w379) -> ("state"=w389:refnum<user-event>, "Filter Wheel ref"=w384:refnum<class "Filter Wheel.lvclass">, "Move"=w395:T9, "Filter Wheel Info"=w394:T7)
            n225 = property on="Tab Control" class="TabCtl (strict)"() -> ("Pages"=w393:refnum<vi>[])  [unwired: 2 in, 2 out]
            n226 = Index Array(array=w393, index=0) -> (element=w391:refnum<vi>)
            n227 = Get Date/Time In Seconds() -> (seconds since 1Jan1904=w381:timestamp)
            n228 = property class="Page"(reference=w391, "PageEnb"=T18."Page Disabled & Grayed" ("Page Enabled State")) -> ()  [unwired: 1 in, 2 out]
            n229 = Bundle By Name(cluster=w379, "Period"=1.0, "next poll"=w381) -> (w380:T13)
            n230 = call "Filter Wheel Validate Move Command.vi"("Filter Wheel Info"=w394, "Move"=w395) -> ("error out"=w385:errorcluster, "Move dup"=w383:T9)  [unwired: 7 in, 1 out]
            n231 = case shown="No Error" w385 {
              selector: w385 -> [_ w413]
              tunnel: w389 -> [w411 w419]
              tunnel: w380 -> [w406 w417]
              tunnel: [w407 w416] -> w388
              tunnel: [w397 w414] -> w387
              tunnel: w384 -> [w410 _]
              tunnel: w383 -> [w409 _]
              frame No Error {
                n232 = Unbundle By Name(w409) -> ("Wheel ID"=w399:i32, "Position"=w398:i32)
                n233 = call-dynamic "Write Wheel Run State.vi"("Run"=TRUE, "Wheel"=w399, "Filter Wheel in"=w410) -> ("Filter Wheel out"=w402:refnum<class "Filter Wheel.lvclass">)  [unwired: 7 in, 1 out]
                n234 = Generate User Event(user event=w411, event data cluster="send data" ("event data")) -> (user event out=w404:refnum<user-event>)  [unwired: 2 in, 1 out]
                n235 = call-dynamic "Get Status.vi"("Filter Wheel in"=w402) -> ("FW Status"=w396:T11, "Filter Wheel out"=w401:refnum<class "Filter Wheel.lvclass">)  [unwired: 8 in, 1 out]
                n236 = Generate User Event(user event=w404, event data cluster="Move Finish" ("event data")) -> ()  [unwired: 2 in, 2 out]
                n237 = Bundle By Name(cluster=w406, "Filter Wheel ref"=w401, "FW Status"=w396) -> (w407:T13)
                n238 = Format Into String(format string="Initiating filter wheel %d move to position %d.", w399, w398) -> (resulting string=w397:string)  [unwired: 2 in, 1 out]
              }
              frame Error {
                n239 = Generate User Event(user event=w419, event data cluster="Error" ("event data")) -> ()  [unwired: 2 in, 2 out]
                n240 = Unbundle By Name(w413) -> ("source"=w412:string)
                n241 = Format Into String(format string="Filter Wheel Move Error: %s", w412) -> (resulting string=w414:string)  [unwired: 2 in, 1 out]
                n242 = Bundle By Name(cluster=w417, "error"=w413, "Error State"=w414) -> (w416:T13)
              }
            }
            n243 = property on="Moving Message" class="Str"("Visible"=w386, "Blinking"=w386) -> ()  [unwired: 2 in, 2 out]
            n244 = call "CC System Message.vi"("Message"=w387) -> ()  [unwired: 10 in, 1 out]
          }
          frame "Move Finish" {
            w432 = FALSE ("Visible")
            n245 = Unbundle By Name(w437) -> ("state"=w439:refnum<user-event>, "Filter Wheel ref"=w442:refnum<class "Filter Wheel.lvclass">, "Move"=w431:T9)
            n246 = property on="Tab Control" class="TabCtl (strict)"() -> ("Pages"=w430:refnum<vi>[])  [unwired: 2 in, 2 out]
            n247 = local read "Last Move Positions"() -> (w423:u32[])
            n248 = Unbundle By Name(w431) -> ("Wheel ID"=w421:i32, "Position"=w440:i32)
            n249 = Index Array(array=w430, index=0) -> (element=w428:refnum<vi>)
            n250 = call-dynamic "Set One Filter.vi"("Position (0:4)"=w440, "Filter Wheel (0:n-1)"=w421, "Filter Wheel in"=w442) -> ("error out"=w424:errorcluster, "Target Counts"=w420:i32, "Filter Wheel out"=w427:refnum<class "Filter Wheel.lvclass">, "Message"=w435:string)  [unwired: 3 in, 2 out]
            n251 = Replace Array Subset(array=w423, new element=w420, index=w421) -> (→"Last Move Positions":u32[])
            n252 = call-dynamic "Write Wheel Run State.vi"("Run"=FALSE, "Wheel"=w421, "Filter Wheel in"=w427) -> ("Filter Wheel out"=w425:refnum<class "Filter Wheel.lvclass">)  [unwired: 7 in, 1 out]
            n253 = case shown="Error .." w424 {
              selector: w424 -> [_ w456]
              tunnel: w439 -> [_ w459]
              tunnel: w437 -> [w448 w457]
              tunnel: [w446 w455] -> w438
              tunnel: w428 -> [w449 w454]
              tunnel: [w449 w454] -> w436
              tunnel: w425 -> [w447 w450]
              tunnel: w435 -> [w444 w452]
              tunnel: ["Move complete." ("string") w451] -> w434
              frame No Error {
                n254 = call "CC System Message.vi"("Message"=w444) -> ()  [unwired: 10 in, 1 out]
                n255 = Bundle By Name(cluster=w448, "Filter Wheel ref"=w447, "Period"=30.0) -> (w446:T13)
              }
              frame Error {
                n256 = Generate User Event(user event=w459, event data cluster="Error" ("event data")) -> ()  [unwired: 2 in, 2 out]
                n257 = Format Into String(format string="Filter Wheel Move Error: %s", w452) -> (resulting string=w451:string)  [unwired: 2 in, 1 out]
                n258 = Bundle By Name(cluster=w457, "Filter Wheel ref"=w450, "error"=w456, "Error State"=w451) -> (w455:T13)
              }
            }
            n259 = property class="Page"(reference=w436, "PageEnb"=T18."Page Enabled" ("Page Enabled State")) -> (error out=w433:errorcluster)  [unwired: 1 in, 1 out]
            n260 = property on="Moving Message" class="Str"(error in=w433, "Visible"=w432, "Blinking"=w432) -> ()  [unwired: 1 in, 2 out]
            n261 = call "CC System Message.vi"("Message"=w434) -> ()  [unwired: 10 in, 1 out]
          }
          frame "Home" {
            w477 = TRUE ("Visible")
            n262 = property on="Moving Message" class="Str"("Visible"=w477, "Blinking"=w477) -> (error out=w476:errorcluster)  [unwired: 2 in, 1 out]
            n263 = Unbundle By Name(w460) -> ("state"=w471:refnum<user-event>, "Filter Wheel ref"=w475:refnum<class "Filter Wheel.lvclass">)
            n264 = Format Into String(format string="Home started on wheel %d", "Wheel To Home") -> (resulting string=w479:string)  [unwired: 2 in, 1 out]
            n265 = call "CC System Message.vi"("error in (no error)"=w476, "Message"=w479) -> ("error out"=w472:errorcluster)  [unwired: 9 in]
            n266 = Get Date/Time In Seconds() -> (seconds since 1Jan1904=w462:timestamp)
            n267 = call-dynamic "Write Wheel Run State.vi"("error in (no error)"=w472, "Run"=TRUE, "Wheel"="Wheel To Home", "Filter Wheel in"=w475) -> ("error out"=w464:errorcluster, "Filter Wheel out"=w467:refnum<class "Filter Wheel.lvclass">)  [unwired: 6 in]
            n268 = Generate User Event(user event=w471, event data cluster="send data" ("event data")) -> (user event out=w470:refnum<user-event>)  [unwired: 2 in, 1 out]
            n269 = Bundle By Name(cluster=w460, "Period"=1.0, "next poll"=w462) -> (w461:T13)
            n270 = call-dynamic "Get Status.vi"("error in (no error)"=w464, "Filter Wheel in"=w467) -> ("FW Status"=w465:T11, "Filter Wheel out"=w466:refnum<class "Filter Wheel.lvclass">)  [unwired: 7 in, 1 out]
            n271 = Generate User Event(user event=w470, event data cluster="Home Finish" ("event data")) -> ()  [unwired: 2 in, 2 out]
            n272 = Bundle By Name(cluster=w461, "Filter Wheel ref"=w466, "FW Status"=w465) -> (w478:T13)
          }
          frame "Home Finish" {
            w486 = FALSE ("Visible")
            n273 = local read "Wheel To Home"() -> (w482:u16)
            n274 = Unbundle By Name(w488) -> ("state"=w489:refnum<user-event>, "Filter Wheel ref"=w492:refnum<class "Filter Wheel.lvclass">)
            n275 = call-dynamic "Home Filter Wheel.vi"("Motor"=w482, "Filter Wheel in"=w492) -> ("error out"=w490:errorcluster, "Log"=w491:string, "Filter Wheel out"=w484:refnum<class "Filter Wheel.lvclass">)  [unwired: 6 in, 1 out]
            n276 = call "CC System Message.vi"("Message"=w491) -> ("error out"=w485:errorcluster)  [unwired: 10 in]
            n277 = call-dynamic "Write Wheel Run State.vi"("Run"=FALSE, "Wheel"=w482, "Filter Wheel in"=w484) -> ("Filter Wheel out"=w483:refnum<class "Filter Wheel.lvclass">)  [unwired: 7 in, 1 out]
            n278 = case shown="Error .." w490 {
              selector: w490 -> [_ w501]
              tunnel: w489 -> [_ w499]
              tunnel: w488 -> [w494 w502]
              tunnel: [w495 w500] -> w487
              tunnel: w483 -> [w496 _]
              frame No Error {
                n279 = Bundle By Name(cluster=w494, "Filter Wheel ref"=w496, "Period"=30.0) -> (w495:T13)
              }
              frame Error {
                n280 = Generate User Event(user event=w499, event data cluster="Error" ("event data")) -> ()  [unwired: 2 in, 2 out]
                n281 = Bundle By Name(cluster=w502, "error"=w501, "Error State"="Homing") -> (w500:T13)
              }
            }
            n282 = property on="Moving Message" class="Str"(error in=w485, "Visible"=w486, "Blinking"=w486) -> ()  [unwired: 1 in, 2 out]
          }
          frame "Stop" {
            n283 = Unbundle By Name(w504) -> ("Filter Wheel ref"=w508:refnum<class "Filter Wheel.lvclass">)
            n284 = call-dynamic "Emergency Stop.vi"("Wheel (-1: all)"=-1, "Filter Wheel in"=w508) -> ("Filter Wheel out"=w506:refnum<class "Filter Wheel.lvclass">)  [unwired: 8 in, 1 out]
            n285 = Bundle By Name(cluster=w504, "Filter Wheel ref"=w506) -> (w505:T13)
            n286 = call "CC System Message.vi"("Message"="Filter Wheel stopped by user.") -> ()  [unwired: 10 in, 1 out]
          }
          frame "Poll" {
            # "Request status from hardware"
            n287 = Unbundle By Name(w517) -> ("state"=w516:refnum<user-event>, "Filter Wheel ref"=w511:refnum<class "Filter Wheel.lvclass">)
            n288 = property on="Filter Wheel Displays" class="Clust (strict)"() -> ("Controls[]"=w522:refnum<vi>[])  [unwired: 2 in, 2 out]
            n289 = call-dynamic "Get Status.vi"("Filter Wheel in"=w511) -> ("error out"=w513:errorcluster, "FW Status"=w510:T11, "Filter Wheel out"=w514:refnum<class "Filter Wheel.lvclass">)  [unwired: 8 in]
            n290 = call-dynamic "Read Home State.vi"("Filter Wheel in"=w511) -> ("Home State"=→"Homed":bool[])  [unwired: 8 in, 2 out]
            n291 = Generate User Event(user event=w516, event data cluster="send data" ("event data")) -> ()  [unwired: 2 in, 2 out]
            n292 = Split 1D Array(array=w522, index=8) -> (first subarray=w519:refnum<vi>[], second subarray=w520:refnum<vi>[])
            n293 = Unbundle By Name(w510) -> ("Notch"=→"On the notch":bool[])
            n294 = case shown="No Error" w513 {
              tunnel: w520 -> [w527 _]
              tunnel: w519 -> [w526 _]
              tunnel: w510 -> [w524 _]
              frame No Error {
                n295 = Unbundle By Name(w524) -> ("Positions"=w523:i32[], "Notch"=w525:bool[])
                n296 = call "Filter Wheel Update Status.vi"("FW Status"=w524) -> ()  [unwired: 10 in, 1 out]
                n297 = for {
                  tunnel: w525 -> [w529] mode=indexing
                  tunnel: w523 -> [w530] mode=indexing
                  tunnel: w527 -> [w532] mode=indexing
                  tunnel: w526 -> [w531] mode=indexing
                  n298 = Not(x=w529) -> ()  [unwired: 1 out]
                  n299 = property class="Ctl"(reference=w532, "Value"=w530) -> ()  [unwired: 1 in, 2 out]
                  n300 = property class="Ctl"(reference=w531, "Blinking"=FALSE, "Value"=w530) -> ()  [unwired: 1 in, 2 out]
                }
              }
              frame Error {
              }
            }
            n301 = Bundle By Name(cluster=w517, "Filter Wheel ref"=w514, "FW Status"=w510) -> (w518:T13)
          }
          frame "send raw string" {
            n302 = Unbundle By Name(w533) -> ("Filter Wheel ref"=w537:refnum<class "Filter Wheel.lvclass">)
            n303 = call-dynamic "Send Raw String.vi"("Cmd String"="Command Preview", "Filter Wheel in"=w537) -> ("Filter Wheel out"=w535:refnum<class "Filter Wheel.lvclass">)  [unwired: 8 in, 1 out]
            n304 = Bundle By Name(cluster=w533, "Filter Wheel ref"=w535) -> (w534:T13)
          }
          frame "read raw" {
            n305 = Unbundle By Name(w541) -> ("Filter Wheel ref"=w540:refnum<class "Filter Wheel.lvclass">)
            n306 = call-dynamic "Read Raw String.vi"("Filter Wheel in"=w540) -> ("Raw String"=→"Response":string, "Filter Wheel out"=w539:refnum<class "Filter Wheel.lvclass">)  [unwired: 8 in, 1 out]
            n307 = Bundle By Name(cluster=w541, "Filter Wheel ref"=w539) -> (w542:T13)
          }
          frame "Send Config" {
            n308 = Unbundle By Name(w548) -> ("Data Q"=w547:refnum<queue>, "Filter Wheel Info"=w544:T7)
            n309 = Bundle By Name(cluster=T16 {"Source"="", "Type"="", "Data"=variant} ("element"), "Source"="Filter Wheel Config" ("Data Type"), "Data"=w544) -> (w543:T16)
            n310 = Enqueue Element(queue=w547, element=w543) -> ()  [unwired: 2 in, 3 out]
          }
          frame "Send Status" {
            n311 = Unbundle By Name(w555) -> ("Data Q"=w554:refnum<queue>, "Filter Wheel ref"=w550:refnum<class "Filter Wheel.lvclass">)
            n312 = call-dynamic "Get Status.vi"("Filter Wheel in"=w550) -> ("FW Status"=w549:T11)  [unwired: 8 in, 2 out]
            n313 = Bundle By Name(cluster=T16 {"Source"="", "Type"="", "Data"=variant} ("element"), "Source"="Filter Wheel Status" ("Data Type"), "Data"=w549) -> (w551:T16)
            n314 = Enqueue Element(queue=w554, element=w551) -> ()  [unwired: 2 in, 3 out]
          }
          frame "Error" {
            w562 = "Filter Wheel" ("Source")
            n315 = Unbundle By Name(w560) -> ("error.status"=w569:bool, "Data Q"=w565:refnum<queue>, "Error State"=w557:string)
            n316 = Bundle By Name(cluster=T19 {"Measured Value"=0.0, "Alarm Low"=0.0, "Alarm High"=0.0, "Message"="", "Source"=""} ("element"), "Source"=w562, "Message"=w557) -> (w563:T19)
            n317 = property on="Error" class="Bool (strict)"("Value"=w569) -> ()  [unwired: 2 in, 2 out]
            n318 = Bundle By Name(cluster=T16 {"Source"="", "Type"="", "Data"=variant} ("element"), "Source"=w562, "Type"="Alarm Set", "Data"=w563) -> (w566:T16)
            n319 = Format Into String(format string="Filter Wheel Error: %s", w557) -> (resulting string=w556:string)  [unwired: 2 in, 1 out]
            n320 = Enqueue Element(queue=w565, element=w566) -> ()  [unwired: 2 in, 3 out]
            n321 = Bundle By Name(cluster=w560, "Period"=30.0) -> (w561:T13)
            n322 = call "CC System Message.vi"("Message"=w556) -> ()  [unwired: 10 in, 1 out]
          }
          frame "Ready" {
            w573 = "Filter Wheel" ("Source")
            n323 = Unbundle By Name(w581) -> ("Data Q"=w577:refnum<queue>, "Error State"=w574:string)
            n324 = Bundle By Name(cluster=T19 {"Measured Value"=0.0, "Alarm Low"=0.0, "Alarm High"=0.0, "Message"="", "Source"=""} ("element"), "Source"=w573, "Message"=w574) -> (w575:T19)
            n325 = Bundle By Name(cluster=T16 {"Source"="", "Type"="", "Data"=variant} ("element"), "Source"=w573, "Type"="Alarm Clear", "Data"=w575) -> (w578:T16)
            n326 = Enqueue Element(queue=w577, element=w578) -> (error out=w571:errorcluster)  [unwired: 2 in, 2 out]
            n327 = call "CC System Message.vi"("Message"="Filter Wheel Ready") -> ()  [unwired: 10 in, 1 out]
            n328 = property on="Error" class="Bool (strict)"(error in=w571, "Value"=FALSE ("Error")) -> ()  [unwired: 1 in, 2 out]
          }
          frame "Shutdown" {
            n329 = Unbundle By Name(w584) -> ("Filter Wheel ref"=w583:refnum<class "Filter Wheel.lvclass">)
            n330 = call-dynamic "Close.vi"("Filter Wheel in"=w583) -> ()  [unwired: 9 in, 2 out]
            n331 = call "CC System Message.vi"("Message"="Filter Wheel shutdown.") -> ()  [unwired: 10 in, 1 out]
          }
        }
      }
      event "Standalone": Value Change {
        n332 = event-data() -> ("NewVal"=w586:bool)  [unwired: 1 in]
        n333 = property on="Close" class="Bool"("Visible"=w586) -> ()  [unwired: 2 in, 2 out]
      }
      event "Alarms?": Value Change {
        n334 = event-data() -> ()  [unwired: 1 in, 6 out]
        n335 = Unbundle By Name(w589) -> ("Filter Wheel ref"=w592:refnum<class "Filter Wheel.lvclass">)
        n336 = property class="Filter Wheel.lvclass"(reference=w592, "Alarms_"="Alarms?") -> (reference out=w590:refnum<class "Filter Wheel.lvclass">)  [unwired: 1 in, 1 out]
        n337 = Bundle By Name(cluster=w589, "Filter Wheel ref"=w590) -> (w588:T13)
      }
      event "Focus Offsets": Value Change {
        n338 = event-data() -> ()  [unwired: 1 in, 6 out]
        n339 = Fract/Exp String To Number(string="Focus Offsets") -> (number=w594:dbl[][])  [unwired: 3 in, 1 out]
        n340 = Number To Fractional String(number=w594, precision (6)=i16 3) -> (F-format string=w595:string[][])  [unwired: 2 in]
        n341 = local write "Focus Offsets"(w595) -> ()
        n342 = call "Rd Wr settings json Filter Wheel Offsets.vi"("Write? (F:Read)"=TRUE, "Offsets"=w594) -> ()  [unwired: 8 in, 2 out]
      }
      event "Open Arduino Log": Value Change {
        n343 = event-data() -> ()  [unwired: 1 in, 6 out]
        n344 = Unbundle By Name(w604) -> ()  [unwired: 1 out]
        n345 = call <vilib>:"Dflt Data Dir.vi"() -> ("App:Default Data Directory"=w603:path)
        n346 = Build Path(base path=w603, name or relative path="Logs") -> (appended path=w601:path)
        n347 = Build Path(base path=w601, name or relative path="Filter Wheel") -> (appended path=w599:path)
        n348 = call <vilib>:"Show in File System.vi"("file or directory path"=w599) -> ()  [unwired: 10 in, 1 out]
      }
      event "Filter Wheel Table": Value Change {
        n349 = event-data() -> ()  [unwired: 1 in, 6 out]
        n350 = call "Rd Wr settings json Filter Wheel Table.vi"("Write? (F:Read)"=TRUE, "Filter Wheel Table"="Filter Wheel Table") -> ()  [unwired: 8 in, 2 out]
      }
      event "Read": Value Change {
        n351 = event-data() -> ()  [unwired: 1 in, 6 out]
        n352 = Unbundle By Name(w610) -> ("state"=w609:refnum<user-event>)
        n353 = Generate User Event(user event=w609, event data cluster="read raw" ("event data")) -> ()  [unwired: 2 in, 2 out]
      }
      event "Error": Value Change {
        n354 = event-data() -> ()  [unwired: 1 in, 6 out]
        n355 = Unbundle By Name(w612) -> ("Error State"=w613:string, "error.code"=w620:i32, "error.source"=w619:string, "error.status"=w618:bool)
        n356 = Format Into String(format string="An error occurred during %s. \nError Number: %d\nError message: %s", w613, w620, w619) -> (resulting string=w617:string)  [unwired: 2 in, 1 out]
        n357 = call "Display Message to User"("Enable"=w618, "Message"=w617) -> ("error out"=w614:errorcluster, "Close"=w616:bool)  [unwired: 8 in]
        n358 = Unbundle By Name(w612) -> ("state"=w611:refnum<user-event>)
        n359 = case shown="True" w616 {
          selector: w616 -> [w622 _]
          tunnel: w612 -> [w625 w628]
          tunnel: [w623 w628] -> w615
          tunnel: w614 -> [w624 _]
          tunnel: w611 -> [_ w627]
          frame False {
            n360 = property on="Error" class="Bool (strict)"("Value"=w622) -> ()  [unwired: 2 in, 2 out]
            n361 = Bundle By Name(cluster=w625, "error"=w624) -> (w623:T13)
          }
          frame True {
            n362 = Generate User Event(user event=w627, event data cluster="Ready" ("event data")) -> ()  [unwired: 2 in, 2 out]
          }
        }
      }
      event Value Change {
        n363 = event-data() -> ()  [unwired: 1 in, 6 out]
        n364 = Unbundle By Name(w634) -> ("Filter Wheel ref"=w637:refnum<class "Filter Wheel.lvclass">, "Name"=w629:string)
        n365 = call "Rd Wr Filter Wheel Settings.vi"("Wheel Name"=w629) -> ("Filter Wheel Settings"=w633:T7)  [unwired: 9 in, 1 out]
        n366 = call-dynamic "Write Homing.vi"("Homing"="Movement Parameters", "Filter Wheel in"=w637) -> ("Filter Wheel out"=w636:refnum<class "Filter Wheel.lvclass">)  [unwired: 8 in, 1 out]
        n367 = Bundle By Name(cluster=w633, "Homing Parameters"="Movement Parameters") -> (w631:T7)
        n368 = Bundle By Name(cluster=w634, "Filter Wheel ref"=w636) -> (w635:T13)
        n369 = call "Rd Wr Filter Wheel Settings.vi"("Wheel Name"=w629, "Write? (F:Read)"=TRUE, "Filter Wheel Settings"=w631) -> ()  [unwired: 7 in, 2 out]
      }
      event "Default Speed": Value Change {
        n370 = event-data() -> ()  [unwired: 1 in, 6 out]
        n371 = Unbundle By Name(w641) -> ("Filter Wheel ref"=w647:refnum<class "Filter Wheel.lvclass">, "Name"=w638:string)
        n372 = call-dynamic "Read Filter Wheel Info.vi"("Filter Wheel in"=w647) -> ("Filter Wheel Info"=w645:T7, "Filter Wheel out"=w646:refnum<class "Filter Wheel.lvclass">)  [unwired: 8 in, 1 out]
        n373 = Bundle By Name(cluster=w645, "Default Speed"="Default Speed") -> (w639:T7)
        n374 = call-dynamic "Write Filter Wheel Info.vi"("Filter Wheel Info"=w639, "Filter Wheel in"=w646) -> ("Filter Wheel out"=w643:refnum<class "Filter Wheel.lvclass">)  [unwired: 8 in, 1 out]
        n375 = call "Rd Wr Filter Wheel Settings.vi"("Wheel Name"=w638, "Write? (F:Read)"=TRUE, "Filter Wheel Settings"=w639) -> ()  [unwired: 7 in, 2 out]
        n376 = Bundle By Name(cluster=w641, "Filter Wheel ref"=w643) -> (w642:T13)
      }
      event "Home": Value Change {
        n377 = event-data() -> ()  [unwired: 1 in, 6 out]
        n378 = Unbundle By Name(w650) -> ("state"=w649:refnum<user-event>)
        n379 = Generate User Event(user event=w649, event data cluster="Home" ("event data")) -> ()  [unwired: 2 in, 2 out]
      }
      event "Simulate": Value Change {
        n380 = event-data() -> ()  [unwired: 1 in, 6 out]
        n381 = Unbundle By Name(w656) -> ("state"=w655:refnum<user-event>)
        n382 = Select(t="set simulation on" ("event data"), s="Simulate", f="set simulation off" ("event data")) -> (s? t:f=w652:string)
        n383 = Generate User Event(user event=w655, event data cluster=w652) -> ()  [unwired: 2 in, 2 out]
      }
      event "Sim Velocity (steps/sec)": Value Change {
        n384 = event-data() -> ()  [unwired: 1 in, 6 out]
        n385 = Unbundle By Name(w657) -> ("Simulate"=w660:bool, "Filter Wheel ref"=w661:refnum<class "Filter Wheel.lvclass">)
        n386 = case shown="True" w660 {
          tunnel: w661 -> [_ w669]
          tunnel: "Sim Velocity (steps/sec)" -> [_ w666]
          tunnel: w657 -> [w662 w665]
          tunnel: [w662 w663] -> w658
          frame False {
          }
          frame True {
            n387 = To More Specific Class(target class=refnum<class "Filter Wheel Simulator.lvclass"> refnum ("Filter Wheel Simulator.lvclass"), reference=w669) -> (specific class reference=w667:refnum<class "Filter Wheel Simulator.lvclass">)  [unwired: 1 in, 1 out]
            n388 = call "Write Velocity (cnts_sec).vi"("Velocity (cnts/sec)"=w666, "Filter Wheel Simulator in"=w667) -> ("Filter Wheel Simulator out"=w664:refnum<class "Filter Wheel Simulator.lvclass">)  [unwired: 8 in, 1 out]
            n389 = Bundle By Name(cluster=w665, "Filter Wheel ref"=w664) -> (w663:T13)
          }
        }
      }
      event "Connect": Value Change {
        n390 = event-data() -> ()  [unwired: 1 in, 6 out]
        n391 = Unbundle By Name(w672) -> ("state"=w671:refnum<user-event>)
        n392 = Generate User Event(user event=w671, event data cluster="connect" ("event data")) -> ()  [unwired: 2 in, 2 out]
      }
      event Value Change {
        n393 = event-data() -> ()  [unwired: 1 in, 1 out]
        n394 = Unbundle By Name(w675) -> ("state"=w674:refnum<user-event>)
        n395 = Generate User Event(user event=w674, event data cluster="show command" ("event data")) -> ()  [unwired: 2 in, 2 out]
      }
      event "Send Command": Value Change {
        n396 = event-data() -> ()  [unwired: 1 in, 6 out]
        n397 = Unbundle By Name(w678) -> ("state"=w677:refnum<user-event>)
        n398 = Generate User Event(user event=w677, event data cluster="send raw string" ("event data")) -> ()  [unwired: 2 in, 2 out]
      }
      event "MOTOR NUMBER": Value Change {
        n399 = event-data() -> ("NewVal"=w681:u8)  [unwired: 1 in]
        n400 = Bundle By Name(cluster=w679, "Motor #"=w681) -> (w680:T13)
      }
      event "STOP": Value Change {
        n401 = event-data() -> ()  [unwired: 1 in, 6 out]
        n402 = Unbundle By Name(w684) -> ("state"=w683:refnum<user-event>)
        n403 = Generate User Event(user event=w683, event data cluster="Stop" ("event data")) -> ()  [unwired: 2 in, 2 out]
      }
      event Value Change {
        n404 = event-data() -> ()  [unwired: 1 in, 1 out]
        n405 = Unbundle By Name(w687) -> ("state"=w686:refnum<user-event>)
        n406 = Generate User Event(user event=w686, event data cluster="set mode" ("event data")) -> ()  [unwired: 2 in, 2 out]
      }
      event "Filter Wheel Displays": Value Change {
        n407 = event-data() -> ("OldVal"=w695:T3, "NewVal"=w688:T3)  [unwired: 1 in]
        n408 = Unbundle By Name(w696) -> ("state"=w699:refnum<user-event>)
        n409 = Not Equal?(x=w695, y=w688) -> (x != y?=w694:T21)
        n410 = Cluster To Array(cluster=w688) -> (array=w691:i32[])
        n411 = Cluster To Array(cluster=w694) -> (array=w693:bool[])
        n412 = Generate User Event(user event=w699, event data cluster="Move" ("event data")) -> ()  [unwired: 2 in, 2 out]
        n413 = Search 1D Array(1D array=w693, element=TRUE) -> (index of element=w689:i32)  [unwired: 1 in]
        n414 = Index Array(array=w691, index=w689) -> (element=w690:i32)
        n415 = Bundle By Name(cluster=w696, "Move.Wheel ID"=w689, "Move.Position"=w690) -> (w697:T13)
      }
      event "Wheels": Value Change {
        n416 = event-data() -> ("NewVal"=w702:i32)  [unwired: 1 in]
        n417 = Unbundle By Name(w700) -> ("Pos Names"=w705:cluster{"Table":string[][]}[])
        n418 = Index Array(array=w705, index=w702) -> (element=w704:cluster{"Table":string[][]})
        n419 = Unbundle(w704) -> ("Table"=w703:string[][])
        n420 = property on="Positions" class="MCListbox (strict)"("ItemNames"=w703) -> ()  [unwired: 2 in, 2 out]
        n421 = Bundle By Name(cluster=w700, "Wheel"=w702) -> (w701:T13)
      }
      event "Wheels": Edit Cell? {
        n422 = event-data() -> ("String"=w709:string, "Coords"=w708:T10)  [unwired: 1 in]
        n423 = Unbundle By Name(w708) -> ("Column"=w711:i32)
        n424 = Not Equal To 0?(x=w711) -> (x != 0?=w710:bool)
        n425 = Bundle By Name(cluster=w706, "Coords"=w708) -> (w707:T13)
        n426 = event-data("String"=w709, "Discard?"=w710) -> ()  [unwired: 1 in, 1 out]
      }
      event "Wheels": Edit Cell {
        n427 = event-data() -> ("String"=w716:string)  [unwired: 1 in]
        n428 = Unbundle By Name(w713) -> ("FW names"=w717:string[], "Coords.Row"=w712:i32)
        n429 = Replace Array Subset(array=w717, new element=w716, index=w712) -> (w715:string[])
        n430 = Bundle By Name(cluster=w713, "FW names"=w715) -> (w714:T13)
      }
      event "Positions": Edit Cell? {
        n431 = event-data() -> ("String"=w723:string, "Coords"=w720:T10)  [unwired: 1 in, 4 out]
        n432 = Unbundle By Name(w720) -> ("Column"=w724:i32)
        n433 = case shown="1" w724 {
          tunnel: w723 -> [w726 w732]
          tunnel: [w726 w729] -> w722
          tunnel: [FALSE ("status") w727] -> w721
          frame 0, Default {
          }
          frame 1 {
            w731 = "%f" ("format string")
            n434 = Scan From String(format string=w731, input string=w732) -> (error out=w728:errorcluster, output 1=w730:dbl)  [unwired: 3 in, 2 out]
            n435 = Unbundle By Name(w728) -> ("status"=w727:bool)
            n436 = Format Into String(format string=w731, w730) -> (resulting string=w729:string)  [unwired: 2 in, 1 out]
          }
        }
        n437 = Bundle By Name(cluster=w718, "Coords"=w720) -> (w719:T13)
        n438 = event-data("String"=w722, "Discard?"=w721) -> ()  [unwired: 1 in, 1 out]
      }
      event "Positions": Edit Cell {
        n439 = event-data() -> ("String"=w741:string)  [unwired: 1 in, 5 out]
        n440 = Unbundle By Name(w734) -> ("Pos Names"=w739:cluster{"Table":string[][]}[], "Coords"=w733:T10)
        n441 = Unbundle By Name(w733) -> ("Row"=w742:i32, "Column"=w743:i32)
        n442 = Index Array(array=w739, index="Wheels") -> (element=w745:cluster{"Table":string[][]})
        n443 = Unbundle(w745) -> ("Table"=w744:string[][])
        n444 = Replace Array Subset(array=w744, new element=w741, index (row)=w742, index (col)=w743) -> (w740:string[][])
        n445 = Bundle("Table"=w740) -> (w738:cluster{"Table":string[][]})  [unwired: 1 in]
        n446 = Replace Array Subset(array=w739, new element=w738, index="Wheels") -> (w736:cluster{"Table":string[][]}[])
        n447 = Bundle By Name(cluster=w734, "Pos Names"=w736) -> (w735:T13)
      }
      event "Add Pos": Value Change {
        n448 = event-data() -> ()  [unwired: 1 in, 6 out]
        n449 = Unbundle By Name(w756) -> ("Pos Names"=w752:cluster{"Table":string[][]}[], "Wheel"=w751:i32)  [unwired: 1 out]
        n450 = Index Array(array=w752, index=w751) -> (element=w750:cluster{"Table":string[][]})
        n451 = Build Array("Unnamed", "0") -> (w753:string[])
        n452 = Unbundle By Name(w750) -> ("Table"=w747:string[][])
        n453 = Build Array (concatenate)(w747, w753) -> (w746:string[][])
        n454 = Bundle By Name(cluster=w750, "Table"=w746) -> (w749:cluster{"Table":string[][]})
        n455 = property on="Positions" class="MCListbox (strict)"("ItemNames"=w746) -> ()  [unwired: 2 in, 2 out]
        n456 = Replace Array Subset(array=w752, new element=w749, index=w751) -> (w748:cluster{"Table":string[][]}[])
        n457 = Bundle By Name(cluster=w756, "Pos Names"=w748) -> (w757:T13)
      }
      event "Remove Pos": Value Change {
        n458 = event-data() -> ()  [unwired: 1 in, 6 out]
        n459 = Unbundle By Name(w765) -> ("Pos Names"=w759:cluster{"Table":string[][]}[], "Wheel"=w764:i32)
        n460 = Index Array(array=w759, index=w764) -> (element=w761:cluster{"Table":string[][]})
        n461 = Unbundle By Name(w761) -> ("Table"=w763:string[][])
        n462 = Delete From Array(array=w763, index (row)="Positions") -> (array with subset deleted=w758:string[][])  [unwired: 2 in, 1 out]
        n463 = Bundle By Name(cluster=w761, "Table"=w758) -> (w760:cluster{"Table":string[][]})
        n464 = property on="Positions" class="MCListbox (strict)"("ItemNames"=w758) -> ()  [unwired: 2 in, 2 out]
        n465 = Replace Array Subset(array=w759, new element=w760, index=w764) -> (w767:cluster{"Table":string[][]}[])
        n466 = Bundle By Name(cluster=w765, "Pos Names"=w767) -> (w766:T13)
      }
      event "Add Fw": Value Change {
        n467 = event-data() -> ()  [unwired: 1 in, 6 out]
        n468 = Unbundle By Name(w771) -> ("FW names"=w769:string[], "Pos Names"=w770:cluster{"Table":string[][]}[])
        n469 = Array Size(array=w769) -> (size(s)=w768:i32)
        n470 = case shown="0..4" w768 {
          tunnel: w769 -> [_ w790]
          tunnel: [w774 w789] -> w772
          tunnel: w771 -> [w774 w788]
          tunnel: w770 -> [_ w777]
          frame 5, Default {
            n471 = One Button Dialog(message="Maximum of 4 filter wheels") -> ()  [unwired: 1 in, 1 out]
          }
          frame 0..4 {
            w781 = "Unnamed"
            n472 = Build Array (concatenate)(w777, cluster{"Table":string[][]} {"Table"=[]}) -> (w775:cluster{"Table":string[][]}[])
            n473 = property on="Wheels" class="MCListbox (strict)"() -> ("ItemNames"=w782:string[][])  [unwired: 2 in, 2 out]
            n474 = Build Array (concatenate)(w790, w781) -> (w784:string[])
            n475 = Build Array(w781, "0" ("element")) -> (w779:string[])
            n476 = Array Size(array=w784) -> (size(s)=w786:i32)
            n477 = Decrement(x=w786) -> (x-1=w785:i32)
            n478 = Build Array (concatenate)(w782, w779) -> (w778:string[][])
            n479 = property on="Wheels" class="MCListbox (strict)"("ItemNames"=w778) -> (error out=w783:errorcluster)  [unwired: 2 in, 1 out]
            n480 = Bundle By Name(cluster=T10 {"Row"=0, "Column"=0} ("Active Cell:Active Cell"), "Row"=w785) -> (w787:T10)
            n481 = Bundle By Name(cluster=w788, "Filter Wheel Info.Num Wheels"=w786, "FW names"=w784, "Pos Names"=w775) -> (w789:T13)
            n482 = property on="Wheels" class="MCListbox (strict)"(error in=w783, "ActiveCell"=w787, "FocusRow"=w785) -> ()  [unwired: 1 in, 2 out]
          }
        }
      }
      event "Remove Fw": Value Change {
        w796 = 1 ("length")
        n483 = event-data() -> ()  [unwired: 1 in, 6 out]
        n484 = Unbundle By Name(w794) -> ("FW names"=w801:string[], "Pos Names"=w800:cluster{"Table":string[][]}[], "Wheel"=w799:i32, "state"=w793:refnum<user-event>)
        n485 = Generate User Event(user event=w793, event data cluster="Show Tables" ("event data")) -> ()  [unwired: 2 in, 2 out]
        n486 = Delete From Array(array=w801, length=w796, index=w799) -> (array with subset deleted=w798:string[])  [unwired: 1 out]
        n487 = Delete From Array(array=w800, length=w796, index=w799) -> (array with subset deleted=w797:cluster{"Table":string[][]}[])  [unwired: 1 out]
        n488 = Bundle By Name(cluster=w794, "FW names"=w798, "Pos Names"=w797) -> (w795:T13)
      }
      event "Save Button": Value Change {
        # "\"Filter Wheel Settings Simulation\":{\n    \"Addr\":\"\",\n    \"Filters\":[\n      {\n        \"Names\":[\"Y\",\"J\",\"H\",\"Open\"],\n        \"Relative Position\":[1,2,3,4],\n        \"Wheel Name\":\"YJH\"\n      },\n      {\n        \"Names\":[\"Z\",\"Narrow\",\"Dark\",\"Open\"],\n        \"Relative Position\":[1,2,3,4],\n        \"Wheel Name\":\"NarrowBand\"\n      }"
        # "Need to copy data from array to filter wheel info cluster"
        n489 = event-data() -> ()  [unwired: 1 in, 6 out]
        n490 = Unbundle By Name(w805) -> ("state"=w803:refnum<user-event>, "Filter Wheel ref"=w813:refnum<class "Filter Wheel.lvclass">, "Filter Wheel Info"=w810:T7, "FW names"=w812:string[], "Pos Names"=w811:cluster{"Table":string[][]}[])
        n491 = for {
          tunnel: w812 -> [w822] mode=indexing
          tunnel: w811 -> [w821] mode=indexing
          tunnel: [w814] -> w808 mode=indexing
          n492 = Unbundle(w821) -> ("Table"=w818:string[][])
          n493 = Index Array(array=w818, index (col)=0 ("disabled index (col)")) -> (element=w819:string[])  [unwired: 1 in]
          n494 = Index Array(array=w818, index (col)=1 ("disabled index (col)")) -> (element=w816:string[])  [unwired: 1 in]
          n495 = Decimal String To Number(string=w816) -> (number=w815:i32[])  [unwired: 2 in, 1 out]
          n496 = Bundle By Name(cluster=T8 {"Names"=[], "Relative Position"=[], "Wheel Name"=""} ("Cluster"), "Wheel Name"=w822, "Relative Position"=w815, "Names"=w819) -> (w814:T8)
        }
        n497 = Generate User Event(user event=w803, event data cluster="Show Filter Wheels" ("event data")) -> ()  [unwired: 2 in, 2 out]
        n498 = Array Size(array=w808) -> (size(s)=w809:i32)
        n499 = Bundle By Name(cluster=w810, "Num Wheels"=w809, "Filters"=w808) -> (w807:T7)
        n500 = call-dynamic "Write Filter Wheel Info.vi"("Filter Wheel Info"=w807, "Filter Wheel in"=w813) -> ("Filter Wheel out"=w802:refnum<class "Filter Wheel.lvclass">)  [unwired: 8 in, 1 out]
        n501 = Bundle By Name(cluster=w805, "Filter Wheel Info"=w807, "Filter Wheel ref"=w802) -> (w806:T13)
      }
      event "Restore Defaults": Value Change {
        n502 = event-data() -> ()  [unwired: 1 in, 6 out]
        n503 = Unbundle By Name(w825) -> ("state"=w824:refnum<user-event>)
        n504 = Generate User Event(user event=w824, event data cluster="init Prime" ("event data")) -> ()  [unwired: 2 in, 2 out]
      }
      event "Close": Value Change {
        n505 = event-data() -> ()  [unwired: 1 in, 2 out]
        n506 = Unbundle By Name(w829) -> ("state"=w828:refnum<user-event>)
        n507 = Generate User Event(user event=w828, event data cluster="Shutdown" ("event data")) -> ()  [unwired: 2 in, 2 out]
      }
    }
  }
  "Wheel Name" <- "Filter Wheel name"
